vi "Text control 1 v0.4.vi"() -> ()   [LabVIEW 2016]
panel:
  in  "Sample I - Probe 4 (Disabled)":u32(ring)=3 items=["SMU1  ", "SMU2  ", "SMU3  ", "SMU4  ", "SMU5  ", "SMU6  ", "VSU1  ", "VSU2  "]
  in  "Sample I - Source/Common":u32(ring) items=["SMU1  ", "SMU2  ", "SMU3  ", "SMU4  ", "SMU5  ", "SMU6  ", "VSU1  ", "VSU2  "]
  in  "Sample I - Probe 3 (Disabled)":u32(ring)=2 items=["SMU1  ", "SMU2  ", "SMU3  ", "SMU4  ", "SMU5  ", "SMU6  ", "VSU1  ", "VSU2  "]
  in  "Sample I - Drain/Gate":u32(ring)=1 items=["SMU1  ", "SMU2  ", "SMU3  ", "SMU4  ", "SMU5  ", "SMU6  ", "VSU1  ", "VSU2  "]
  in  "Sample - Probe 4":u32(ring)=3 items=["SMU1  ", "SMU2  ", "SMU3  ", "SMU4  ", "SMU5  ", "SMU6  ", "VSU1  ", "VSU2  "]
  in  "Sample - Source/Common":u32(ring) items=["SMU1  ", "SMU2  ", "SMU3  ", "SMU4  ", "SMU5  ", "SMU6  ", "VSU1  ", "VSU2  "]
  in  "Sample - Gate":u32(ring)=2 items=["SMU1  ", "SMU2  ", "SMU3  ", "SMU4  ", "SMU5  ", "SMU6  ", "VSU1  ", "VSU2  "]
  in  "Sample - Drain":u32(ring)=1 items=["SMU1  ", "SMU2  ", "SMU3  ", "SMU4  ", "SMU5  ", "SMU6  ", "VSU1  ", "VSU2  "]
  in  "VSU2 Stress - Source/Common":u32(ring) items=["SMU1  ", "SMU2  ", "SMU3  ", "SMU4  ", "SMU5  ", "SMU6  ", "VSU1  "]
  in  "Stress I - Source/Common":u32(ring) items=["SMU1  ", "SMU2  ", "SMU3  ", "SMU4  ", "SMU5  ", "SMU6  ", "VSU1  ", "VSU2  "]
  in  "Stress I - Drain/Gate":u32(ring)=1 items=["SMU1  ", "SMU2  ", "SMU3  ", "SMU4  ", "SMU5  ", "SMU6  ", "VSU1  ", "VSU2  "]
  in  "Stress V - Source/Common":u32(ring) items=["SMU1  ", "SMU2  ", "SMU3  ", "SMU4  ", "SMU5  ", "SMU6  ", "VSU1  ", "VSU2  "]
  in  "Stress V - Gate":u32(ring)=2 items=["SMU1  ", "SMU2  ", "SMU3  ", "SMU4  ", "SMU5  ", "SMU6  ", "VSU1  ", "VSU2  "]
  in  "Stress V - Drain":u32(ring)=1 items=["SMU1  ", "SMU2  ", "SMU3  ", "SMU4  ", "SMU5  ", "SMU6  ", "VSU1  ", "VSU2  "]
  in  "FPP - Source":u32(ring)=6 items=["SMU1  ", "SMU2  ", "SMU3  ", "SMU4  ", "SMU5  ", "SMU6  ", "VSU1  ", "VSU2  "]
  in  "FPP - Probe 2":u32(ring)=3 items=["SMU1  ", "SMU2  ", "SMU3  ", "SMU4  ", "SMU5  ", "SMU6  ", "VSU1  ", "VSU2  "]
  in  "FPP - Probe 1":u32(ring) items=["SMU1  ", "SMU2  ", "SMU3  ", "SMU4  ", "SMU5  ", "SMU6  ", "VSU1  ", "VSU2  "]
  in  "FPP - Gate":u32(ring)=2 items=["SMU1  ", "SMU2  ", "SMU3  ", "SMU4  ", "SMU5  ", "SMU6  ", "VSU1  ", "VSU2  "]
  in  "FPP - Drain":u32(ring)=1 items=["SMU1  ", "SMU2  ", "SMU3  ", "SMU4  ", "SMU5  ", "SMU6  ", "VSU1  ", "VSU2  "]
  in  "Pulsed Stress V - Gate":u32(ring)=2 items=["SMU1  ", "SMU2  ", "SMU3  ", "SMU4  ", "SMU5  ", "SMU6  ", "VSU1  ", "VSU2  "]
  in  "Pulsed Stress V - Source/Common":u32(ring) items=["SMU1  ", "SMU2  ", "SMU3  ", "SMU4  ", "SMU5  ", "SMU6  ", "VSU1  ", "VSU2  "]
  in  "Pulsed Stress V - Drain":u32(ring)=1 items=["SMU1  ", "SMU2  ", "SMU3  ", "SMU4  ", "SMU5  ", "SMU6  ", "VSU1  ", "VSU2  "]
  in  "Pulsed Stress V - Vextra":u32(ring)=7 items=["SMU1  ", "SMU2  ", "SMU3  ", "SMU4  ", "SMU5  ", "SMU6  ", "VSU1  ", "VSU2  "]
  in  "Pulsed Stress V - Probe 4":u32(ring)=3 items=["SMU1  ", "SMU2  ", "SMU3  ", "SMU4  ", "SMU5  ", "SMU6  ", "VSU1  ", "VSU2  "]
  in  "Transfer/Output - Probe 4":u32(ring)=3 items=["SMU1  ", "SMU2  ", "SMU3  ", "SMU4  ", "SMU5  ", "SMU6  ", "VSU1  ", "VSU2  "]
  in  "Transfer/Output - Source/Common":u32(ring) items=["SMU1  ", "SMU2  ", "SMU3  ", "SMU4  ", "SMU5  ", "SMU6  ", "VSU1  ", "VSU2  "]
  in  "Transfer/Output - Gate":u32(ring)=2 items=["SMU1  ", "SMU2  ", "SMU3  ", "SMU4  ", "SMU5  ", "SMU6  ", "VSU1  ", "VSU2  "]
  in  "Transfer/Output - Drain":u32(ring)=1 items=["SMU1  ", "SMU2  ", "SMU3  ", "SMU4  ", "SMU5  ", "SMU6  ", "VSU1  ", "VSU2  "]
  in  "Panel Controls 2":T1={"Emergency Stop"=refnum, "TransGraph Max"=1e-05, "Text/Graph (text=false)"=TRUE, "TransGraph Min"=1e-11} {"TransGraph Min" format="%.2e"; "TransGraph Max" format="%.2e"}
  out "Currently running:":string="#output s 0 0 0 -0.008 0.008 0.002"
  in  "Lines left to run:":string
  in  "Standby":T2
  in  "Full Reset":bool
  in  "SMU4":cluster{"on/off":bool, "Voltage":dbl} {"Voltage" min=-100.0 max=100.0 format="%.2f"}
  in  "Source/Drain\nRange":u8(slide)=6 max=11 scale=0.0..11.0
  in  "Source/Drain\nRange mode":u16(ring) items=["Auto", "Limited", "Fixed"]
  in  "Gate Range":u8(slide)=6 max=11 scale=0.0..11.0
  in  "Gate Range\nmode":u16(ring) items=["Auto", "Limited", "Fixed"]
  in  "Gate":T3={"Gate Start"=0.0, "Gate Stop"=2.0, "Gate Step (linear only)"=1.0, "Gate Compliance"=0.0001, "Gate PComp"=0.0, "Range mode"=0, "Range"=6} {"Range" max=11 scale=0.0..11.0; "Range mode" items=["Auto", "Limited", "Fixed"]; "Gate PComp" format="%^.2e"; "Gate Compliance" format="%^.2e"; "Gate Step (linear only)" format="%^.4e"; "Gate Stop" format="%^.4e"; "Gate Start" format="%^.4e"}
  in  "Drain 2":T4={"Drain Start"=0.0, "Drain Stop"=2.0, "Drain Compliance"=0.0001, "Drain Step"=1.0, "Drain PComp"=0.0, "Range mode"=0, "Range"=6} {"Range" max=11 scale=0.0..11.0; "Range mode" items=["Auto", "Limited", "Fixed"]; "Drain PComp" format="%^.2e"; "Drain Step" format="%^.4e"; "Drain Compliance" format="%^.2e"; "Drain Stop" format="%^.4e"; "Drain Start" format="%^.4e"}
  in  "Timings 2":T5={"integration time"=0, "Short/Long integration time"=0.00064, "hold time (sec)"=0.0, "delay time (sec)"=0.0, "Step Time (0 disables)"=0.0, "sweep method"=0, "Pulse period"=0.005, "Base voltage"=0.0, "Pulse width"=0.0005} {"Pulse width" min=0.0005 max=0.1 step=0.0001 format="%.4f"; "Base voltage" format="%^.4e"; "Pulse period" min=0.005 max=1.0 step=0.0001 format="%.4f"; "sweep method" items=["Continuous", "Pulsed"]; "Step Time (0 disables)" format="%.2f"; "delay time (sec)" format="%.4f"; "hold time (sec)" format="%.4f"; "Short/Long integration time" format="%^.0e"; "integration time" scale=0.0..2.0}
  in  "Panel Controls":T6={"Emergency Stop"=refnum, "TransGraph Max"=1e-05, "Text/Graph (text=false)"=TRUE} {"TransGraph Max" format="%.2e"}
  in  "Interrupt run":bool
  in  "Drain: Compliance":dbl=0.001 format="%.8f"
  in  "Gate: Compliance":dbl=0.001 format="%.8f"
  out "Path":path=path "C:/users/rlp38/09Apr2009LTtesting/test2.txt"
  in  "hold time /s":dbl format="%.2f"
  in  "delay time /s":dbl format="%.2f"
  in  "integration time":u32(slide)=1 max=2 step=1 scale=0.0..2.0
  in  "Integration time (short)":dbl=0.0019 min=8e-05 max=0.0019 step=8e-05 format="%^.0e"
  in  "Integration time (long)":dbl=0.32 min=0.04 max=2.0 step=0.02 format="%.2f"
  in  "Step delay /s":dbl format="%.2f"
  in  "Program":string="#pulsedstressV d 0.03 20 0 0.5 0.0827 5\n#\n#itime l 0.32\n#gaterangemode a\n#drainrangemode a\n#pulsed on 0.05 0 0.02\n#transfer d -10 40 1 5 40 35\n#transfer d -10 40 1 5 40 35\n#transfer d -10 40 1 5 40 35\n#output d 0 40 20 0 40 1\n#\n#\n#sample 1 0.008 221 6 0.003\n#samplei 400e-6 200 6 0.002 0.1\n#vsu2pulse -10 4\n#\n#stressV 0.016 0.03 2e-4 0.1e-3 11\n#stressI 220e-7 0.08 15\n#transfer s -1 1 0.5 -0.005 0.005 0.005\n#output s 0 0 0 -0.008 0.008 0.002\n"
  # "SMUs"
  # "Syntax:\nitime [s|m|l] time(sec): [s|m|l] determines the integration time setting (small|medium|long) and time sets the value.\nNOTE: The value of the integration time has to be within the range allowed by its category (s|m|l), otherwise, the closest value will be used. (e.g. if the category is set to short but the time value is very long, the actual value used will be the maximum short integration time.\nIntegration times:\n    Short: Default: 640 us. Range: 8E-5 - 1.92E-3 seconds.\n    Medium: Fixed at 1 NPL cycle (0.02 seconds).\n    Long: Default: 16 NPL cycles (0.32 seconds). Range: 2-100 NPL cycles (0.04 seconds - 2 seconds).\ngaterangemode [a|l|f]\ndrainrangemode [a|l|f]\npulsed [on|off] PulsePeriod(sec) PulseBaseVoltage PulseONWidth(sec)\nstandby [on l off]\nwait NumMilliseconds\nwait-min NumMinutes\n# texthere = comment\ntransfer [s|d] VgStart VgStop VgStep VdStart VdStop VdStep\noutput [s|d] VgStart VgStop VgStep VdStart VdStop VdStep\nsample Vg Vd NumSamples Time(s) SampleInterval(s)\nsamplei Idg NumSamples Time(s) SampleInterval(s) VDGcompliance\n# if in doubt use SampleInterval(s) = 0.004\nstressV VG VD IGcompliance IDcompliance Duration(sec)\nstressI IDG VDGcompliance Duration(sec)\nvsu2pulse Bias Duration(s)\npulsedstressV [s|d] VEstop VgON VgOFF Period(s) PulseONwidth(s) Vd\nsample-fpp Vg Vd NumSamples Time\nresample-fpp Vg Vd\ntransfer-fpp [s|d] VgStart VgStop VgStep VdStart VdStop VdStep\noutput-fpp [s|d] VgStart VgStop VgStep VdStart VdStop VdStep"
  # "100 samples is approx 13s with medium integration"
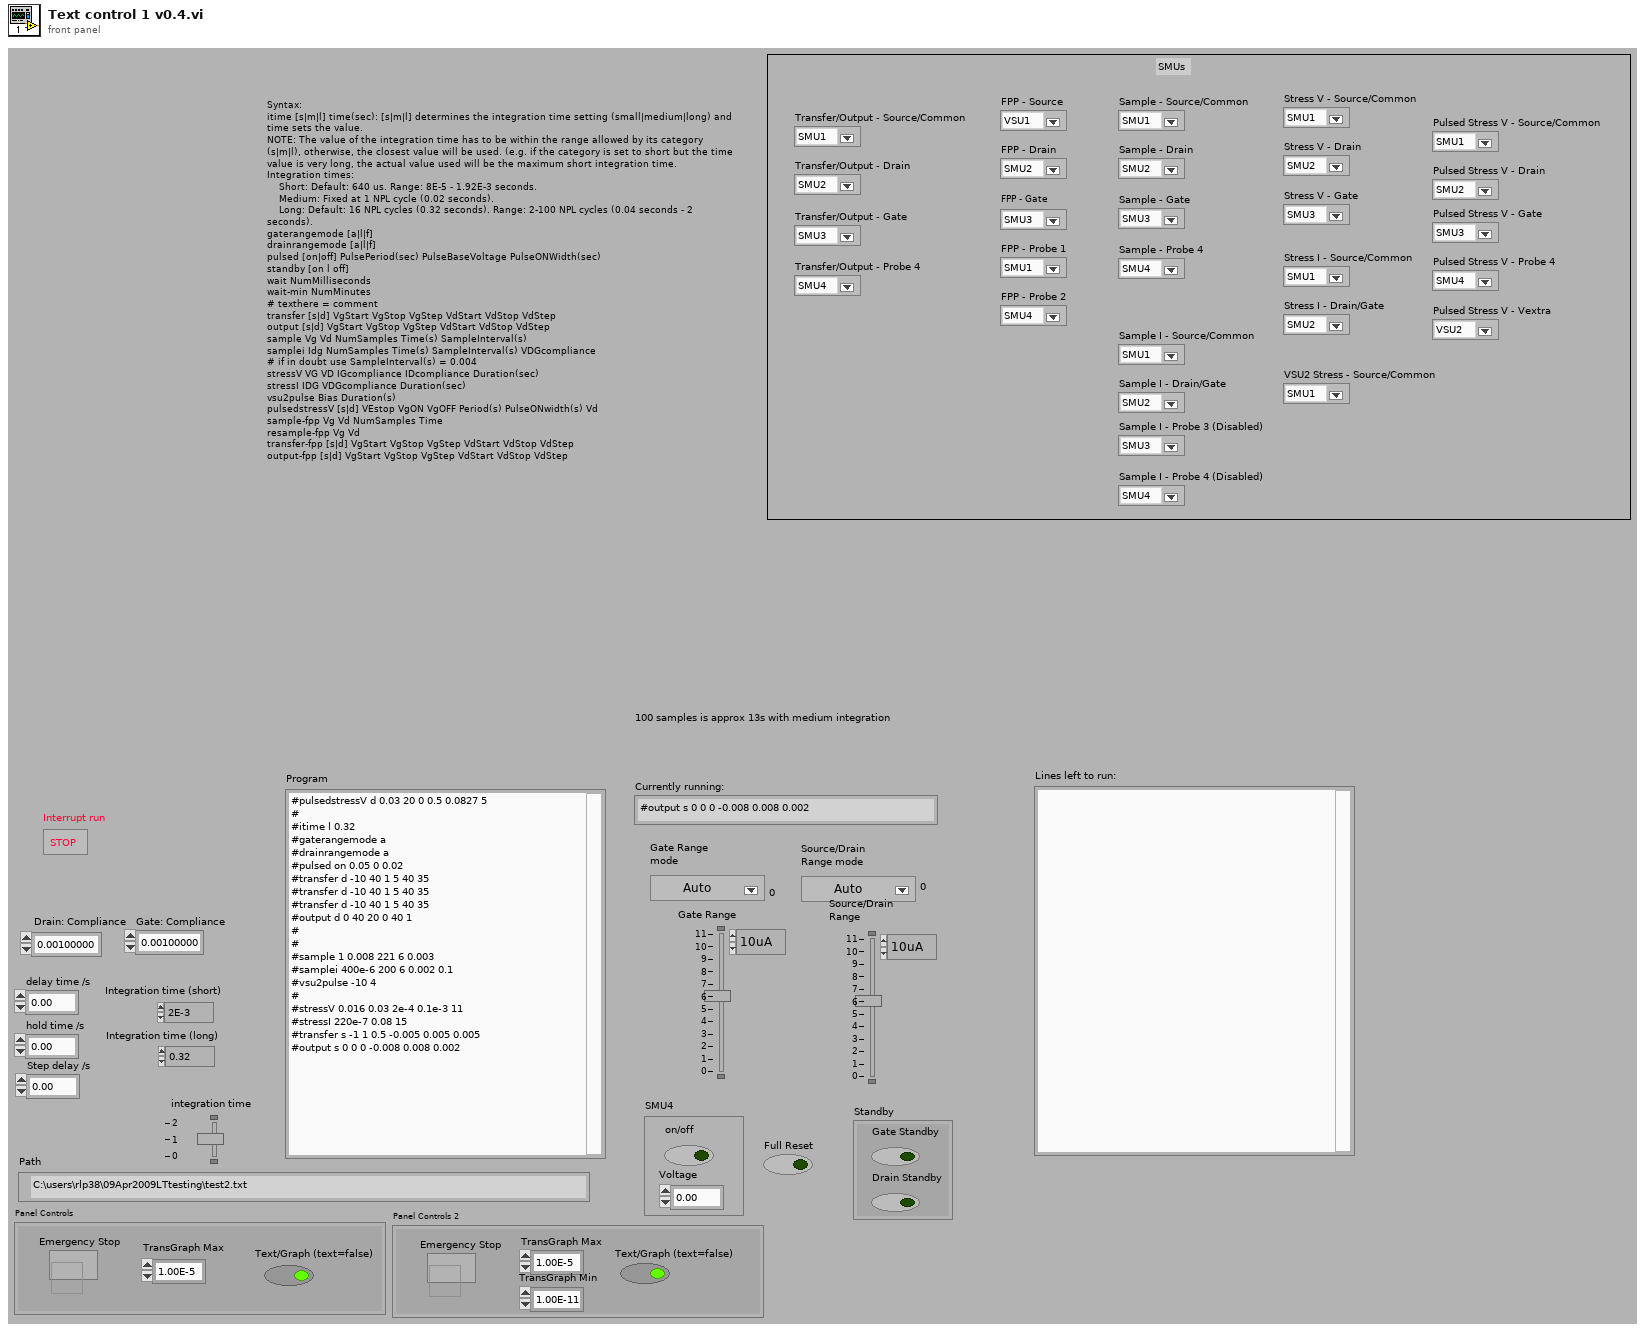
[diagram p1: front panel]
types:
  T1 = cluster{"Emergency Stop":refnum<vi>, "TransGraph Max":dbl, "Text/Graph (text=false)":bool, "TransGraph Min":dbl}
  T2 = cluster{"Gate Standby":bool, "Drain Standby":bool}
  T3 = cluster{"Gate Start":dbl, "Gate Stop":dbl, "Gate Step (linear only)":dbl, "Gate Compliance":dbl, "Gate PComp":dbl, "Range mode":u16, "Range":u8}
  T4 = cluster{"Drain Start":dbl, "Drain Stop":dbl, "Drain Compliance":dbl, "Drain Step":dbl, "Drain PComp":dbl, "Range mode":u16, "Range":u8}
  T5 = cluster{"integration time":u32, "Short/Long integration time":dbl, "hold time (sec)":dbl, "delay time (sec)":dbl, "Step Time (0 disables)":dbl, "sweep method":u16, "Pulse period":dbl, "Base voltage":dbl, "Pulse width":dbl}
  T6 = cluster{"Emergency Stop":refnum<vi>, "TransGraph Max":dbl, "Text/Graph (text=false)":bool}
  T7 = enum16{"open", "replace", "create", "open or create", "replace or create", "replace or create with confirmation"}
  T8 = cluster{"V2 Start":dbl, "V2 Step":dbl, "Number of points":i32}
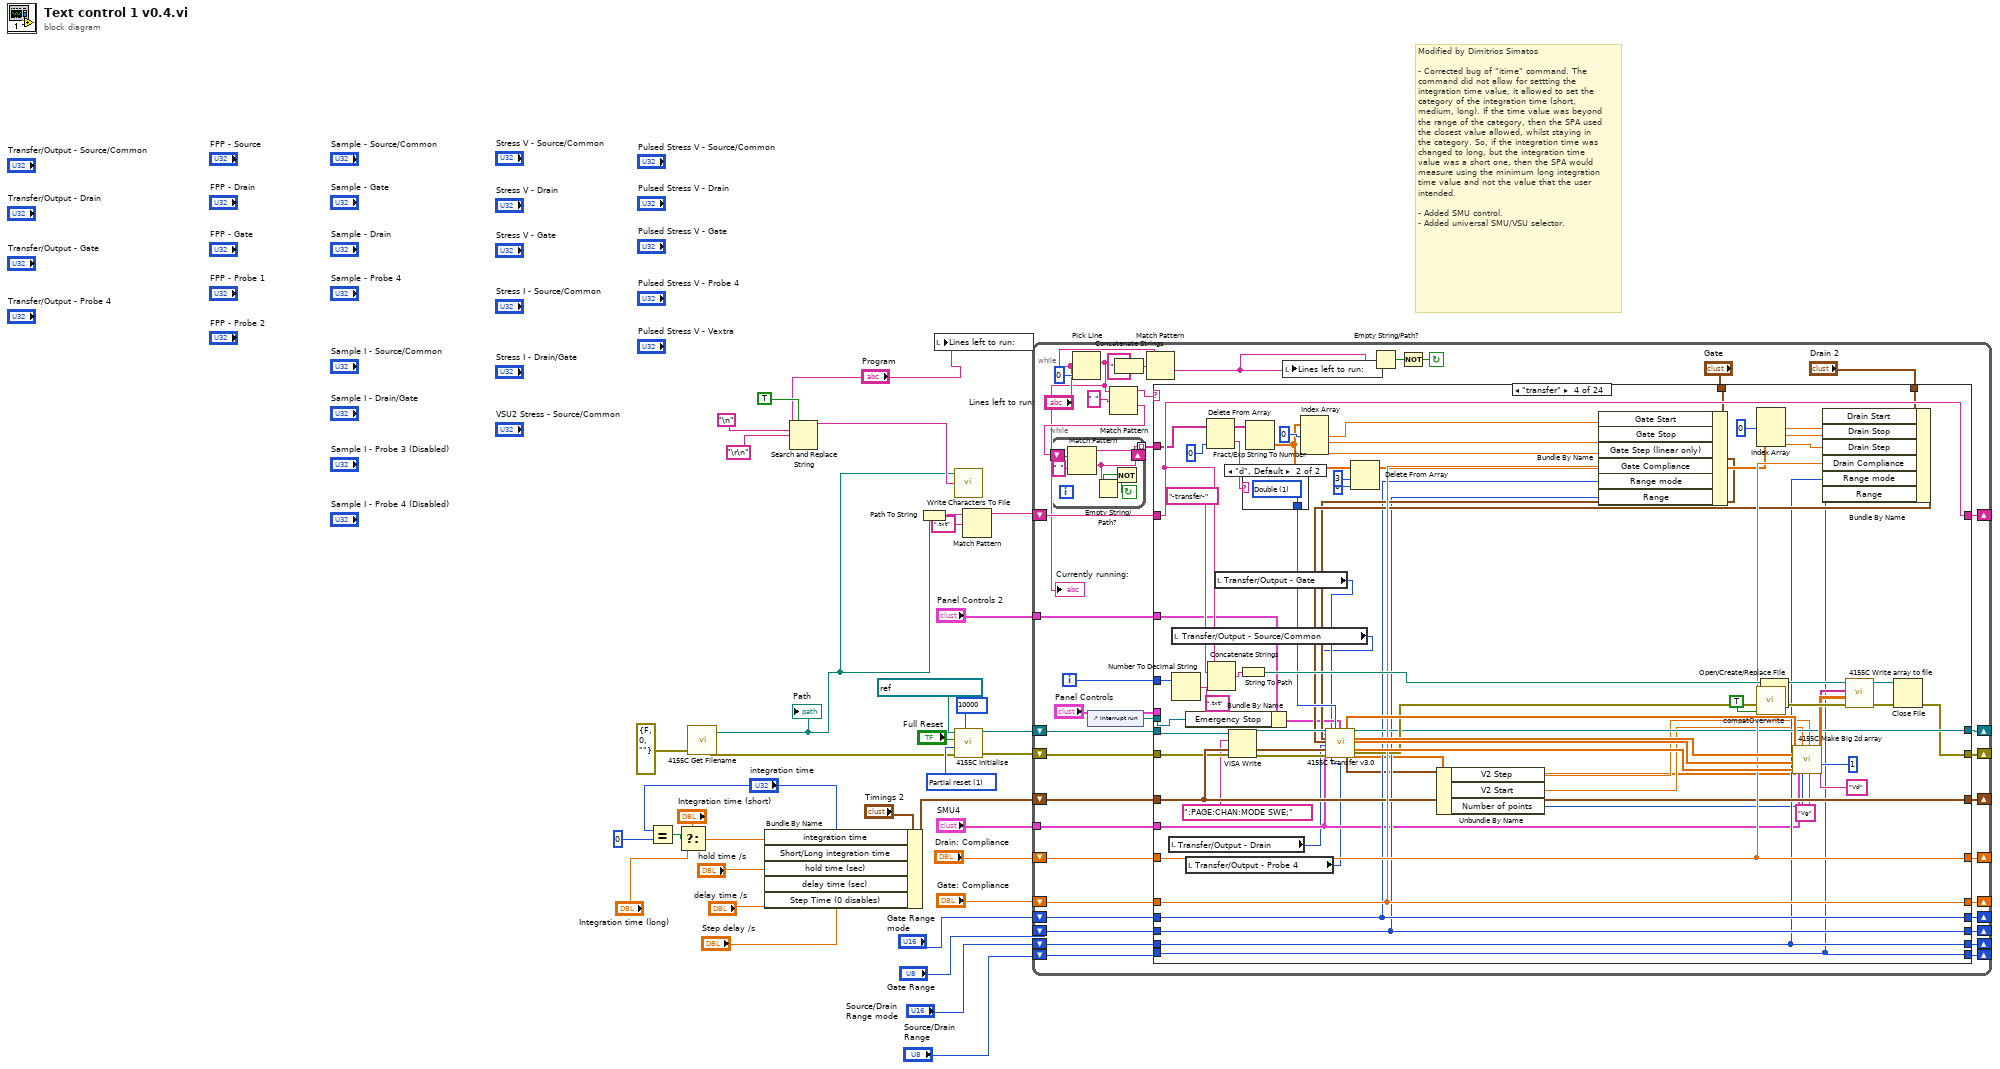
[diagram p0: block diagram]
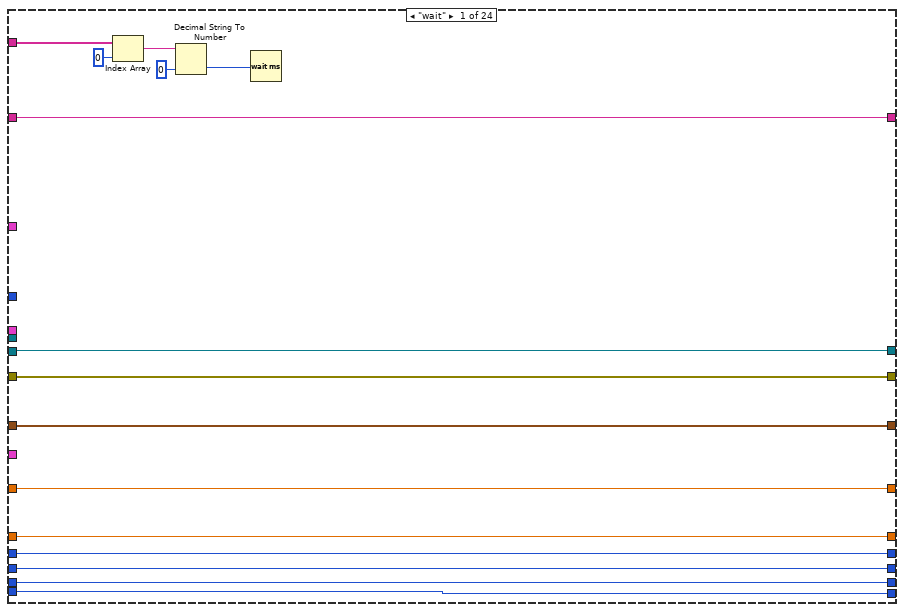
[diagram p2: hidden frame]
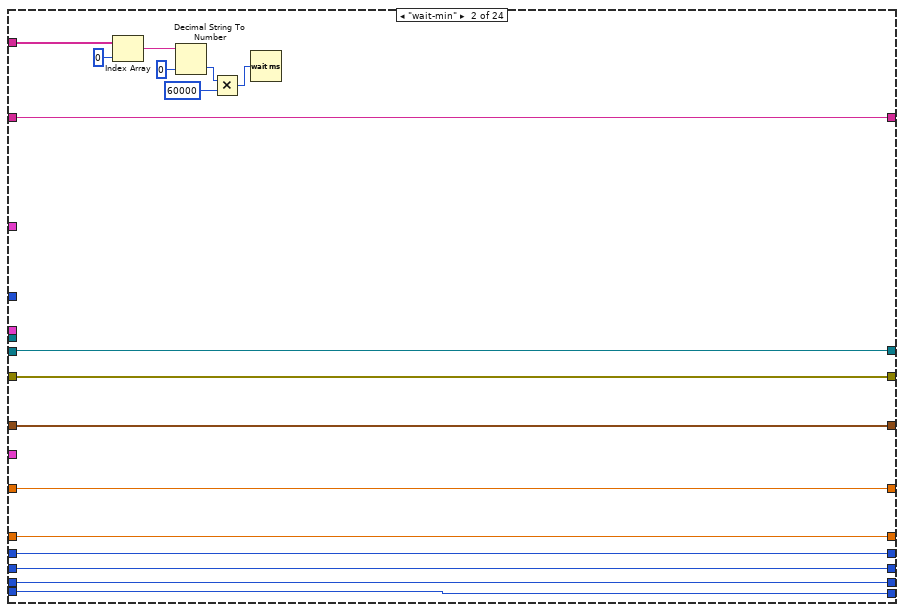
[diagram p3: hidden frame]
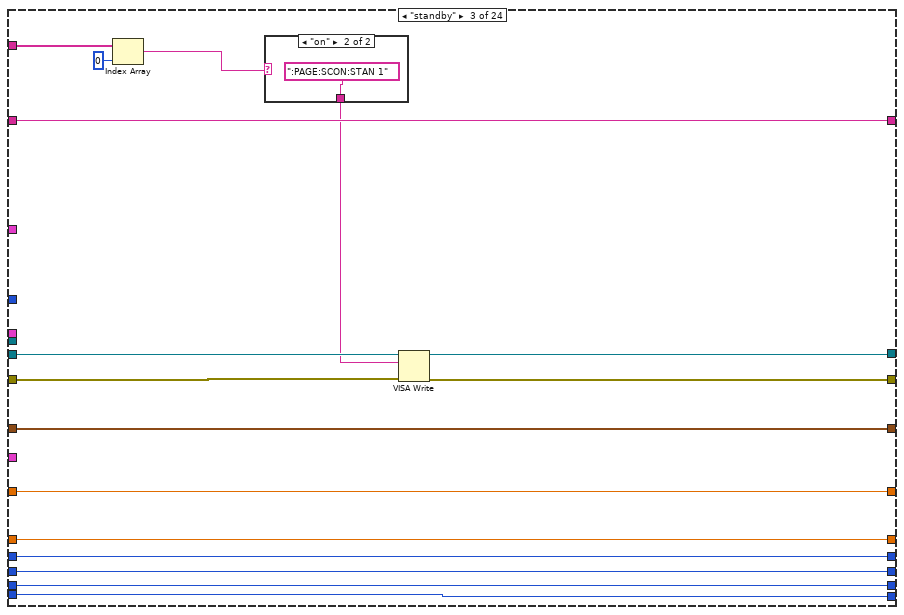
[diagram p4: hidden frame]
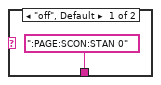
[diagram p5: hidden frame]
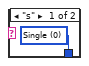
[diagram p6: hidden frame]
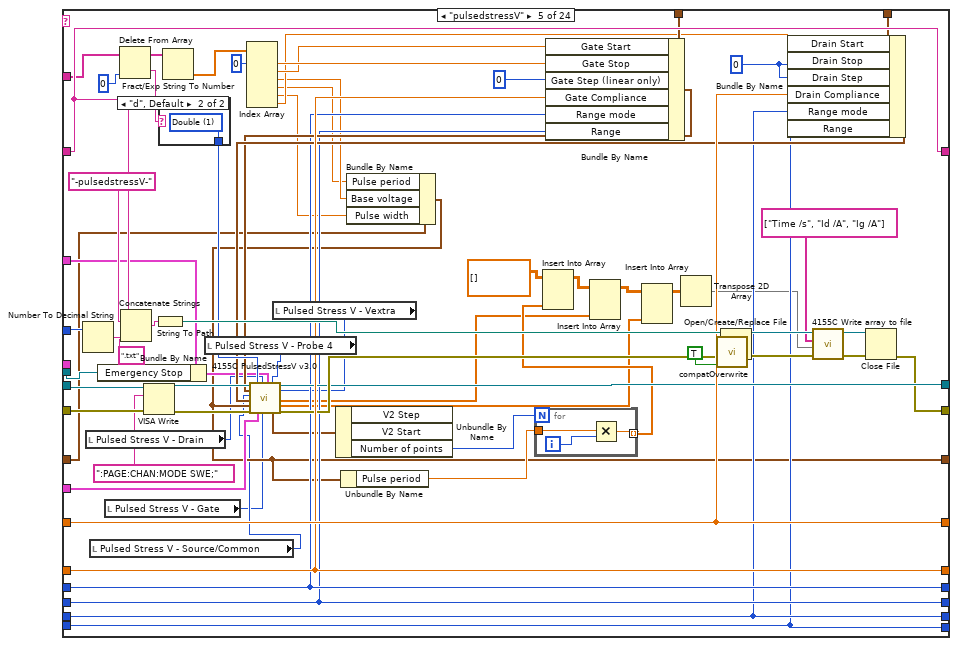
[diagram p7: hidden frame]
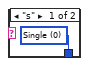
[diagram p8: hidden frame]
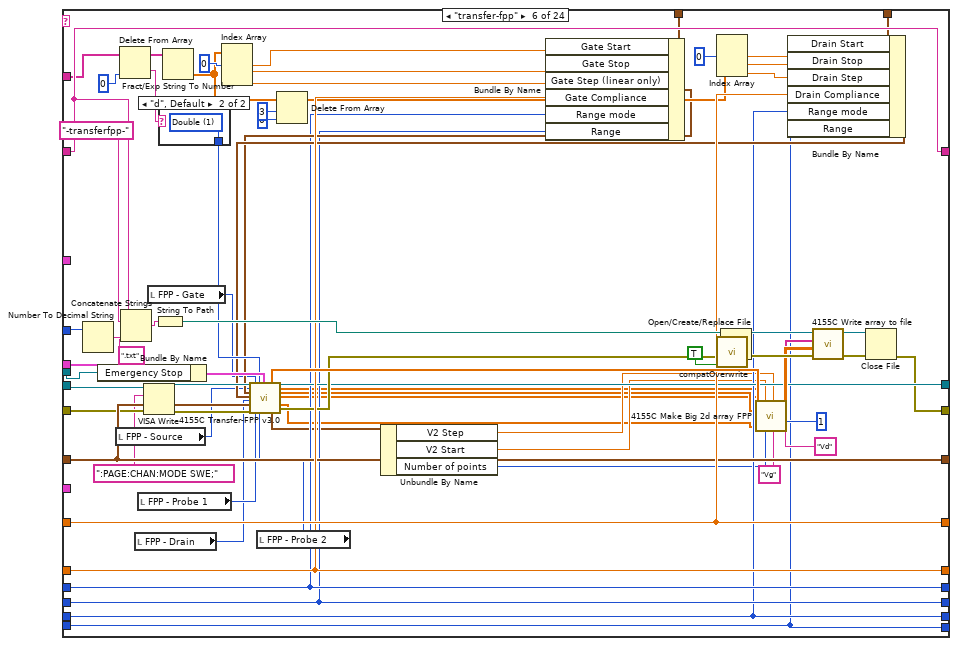
[diagram p9: hidden frame]
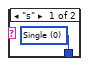
[diagram p10: hidden frame]
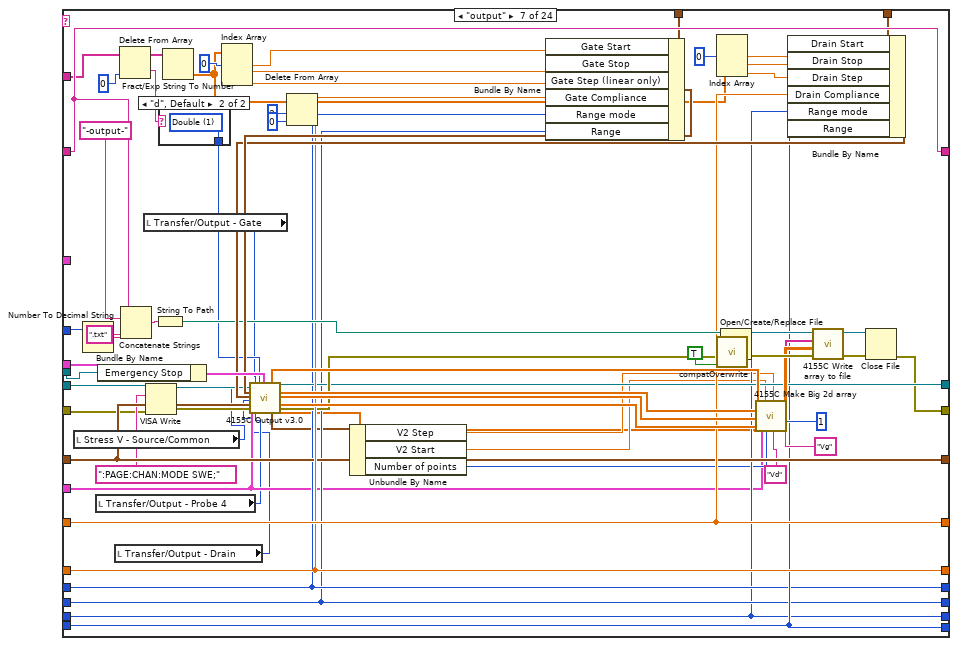
[diagram p11: hidden frame]
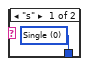
[diagram p12: hidden frame]
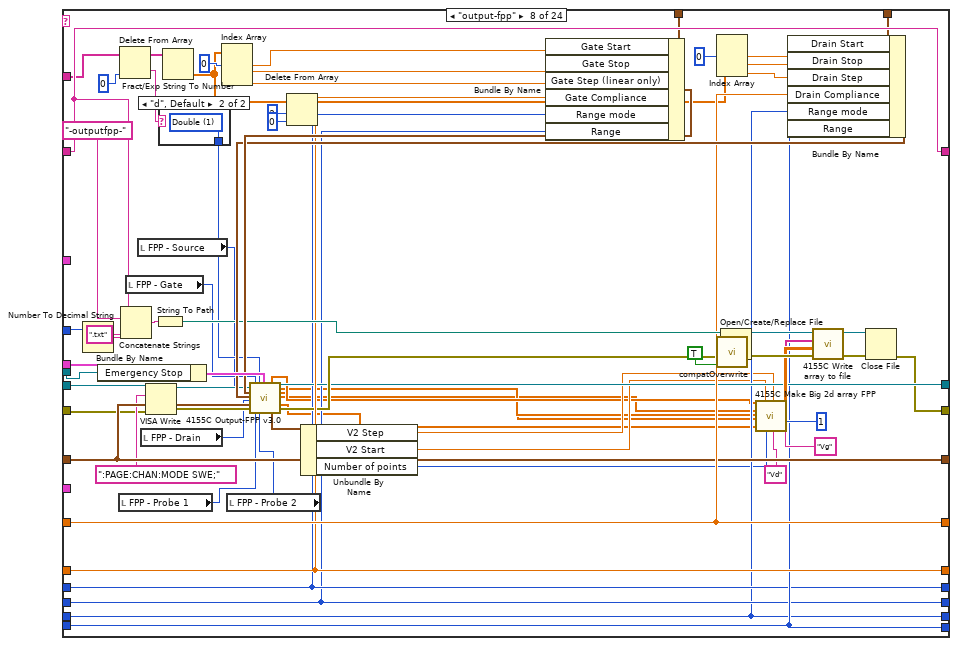
[diagram p13: hidden frame]
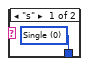
[diagram p14: hidden frame]
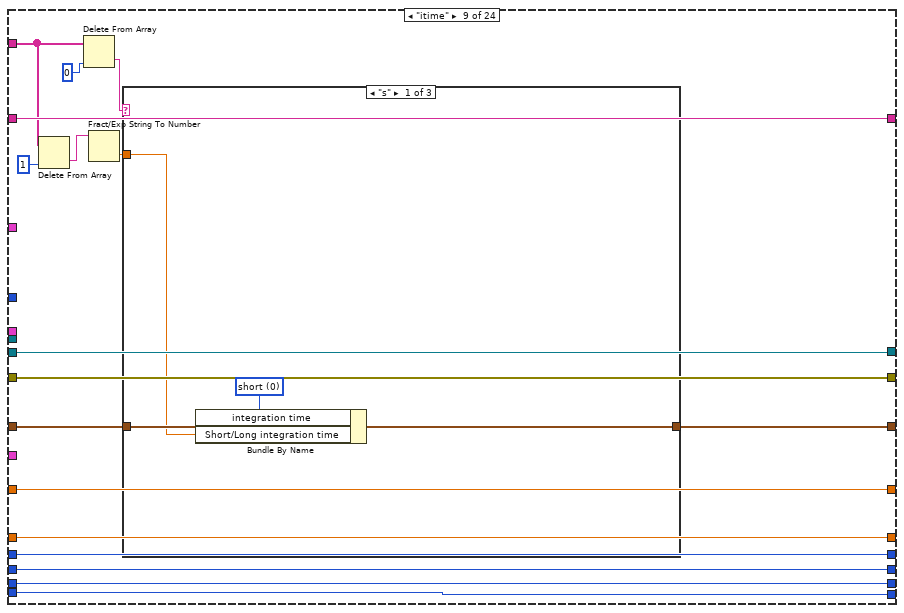
[diagram p15: hidden frame]
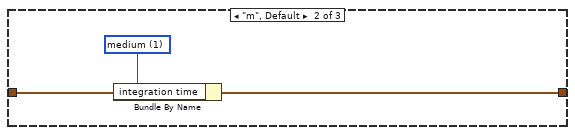
[diagram p16: hidden frame]
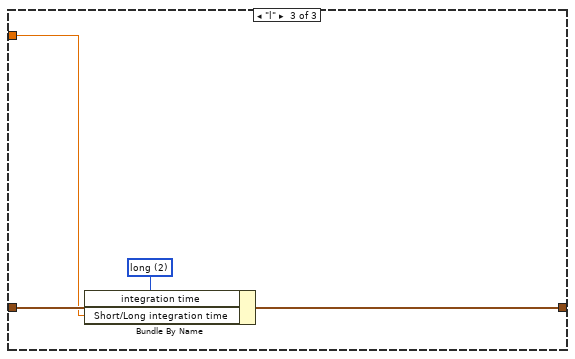
[diagram p17: hidden frame]
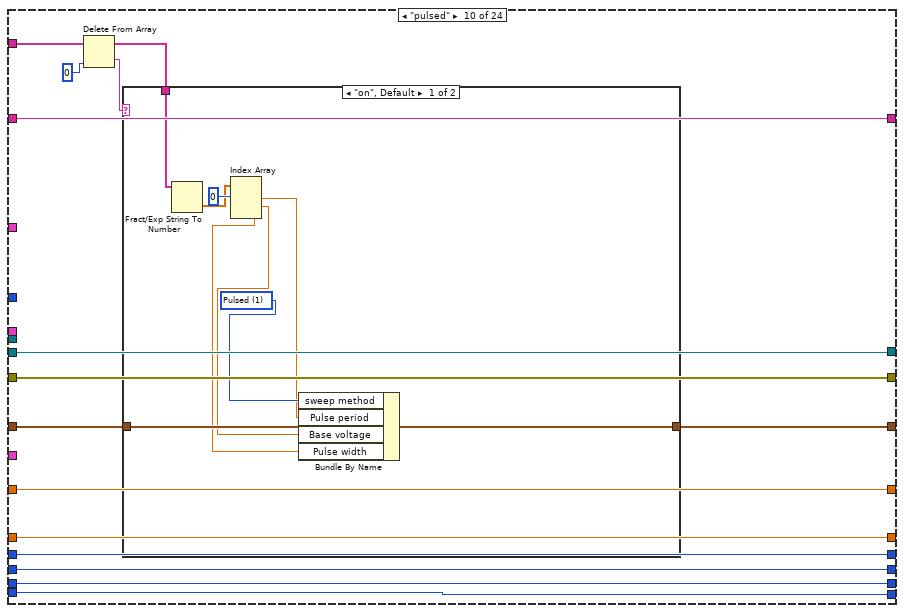
[diagram p18: hidden frame]
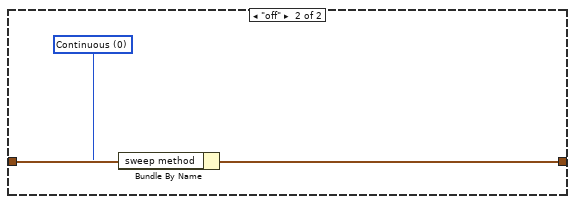
[diagram p19: hidden frame]
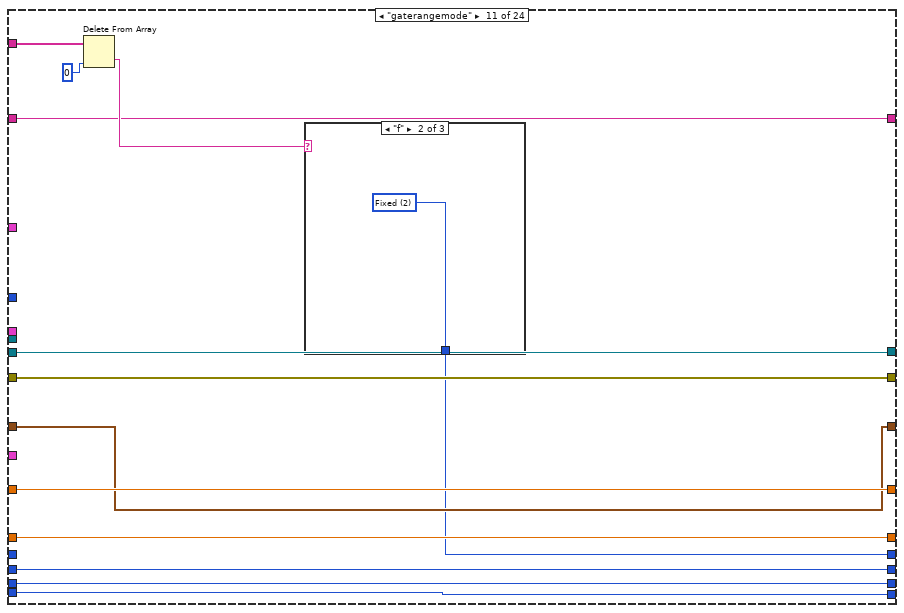
[diagram p20: hidden frame]
diagram:
  w27 = u16 1 items=["Reset All", "Partial reset"] ("Type of reset")
  # "Modified by Dimitrios Simatos\n\n- Corrected bug of \"itime\" command. The command did not allow for settting the integration time value, it allowed to set the category of the integration time (short, medium, long). If the time value was beyond the range of the category, then the SPA used the closest value allowed, whilst staying in the category. So, if the integration time was changed to long, but the integration time value was a short one, then the SPA would measure using the minimum long integration time value and not the value that the user intended.\n\n- Added SMU control.\n- Added universal SMU/VSU selector."
  n1 = Equal?(x="integration time", y=u32 0) -> (x = y?=w31:bool)
  n2 = Select(t="Integration time (short)", s=w31, f="Integration time (long)") -> (s? t:f=w35:dbl)
  n3 = call "4155C Get Filename.vi"("error in (no error)"=errorcluster {"status"=FALSE, "code"=0, "source"=""}) -> ("error out"=w22:errorcluster, "path"=w6:path)  [unwired: 2 in, 1 out]
  "Path" <- w6
  n4 = Bundle By Name(cluster="Timings 2", "integration time"="integration time", "Short/Long integration time"=w35, "hold time (sec)"="hold time /s", "delay time (sec)"="delay time /s", "Step Time (0 disables)"="Step delay /s") -> (w19:T5)
  n5 = Search and Replace String(replace all?=TRUE ("replace all? (F)"), input string="Program", search string="\n", replace string="\r\n") -> (result string=w9:string)  [unwired: 4 in, 3 out]
  n6 = Path To String(path=w6) -> (string=w5:string)
  n7 = local write "Lines left to run:"("Program") -> ()
  n8 = call <vilib>:"Write Characters To File.vi"("character string"=w9, "file path (dialog if empty)"=w6) -> ()  [unwired: 3 in, 1 out]
  n9 = call "4155C Initialise.vi"("VISA resource name in"=refnum<visa-resource-name> "GPIB0::14::INSTR", "Reset"="Full Reset", "Type of reset"=w27, "error in (no error)"=w22, "VISA Timeout Value"=u32 10000) -> ("VISA Resource Name out"=w21:refnum<visa-resource-name>, "error out"=w20:errorcluster)
  n10 = Match Pattern(string=w5, regular expression=".txt") -> (before substring=w4:string)  [unwired: 1 in, 3 out]
  n11 = while {
    tunnel: "SMU4" -> [w41]
    shift-left: "Source/Drain\nRange" -> [w46]
    shift-right: [w42] -> _
    shift-left: "Source/Drain\nRange mode" -> [w47]
    shift-right: [w43] -> _
    shift-left: "Gate Range" -> [w48]
    shift-right: [w44] -> _
    shift-left: "Gate Range\nmode" -> [w49]
    shift-right: [w45] -> _
    shift-left: "Gate: Compliance" -> [w61]
    shift-right: [w55] -> _
    shift-left: "Drain: Compliance" -> [w62]
    shift-right: [w56] -> _
    shift-left: w19 -> [w63]
    shift-right: [w57] -> _
    shift-left: w20 -> [w64]
    shift-right: [w58] -> _
    shift-left: w21 -> [w65]
    shift-right: [w59] -> _
    shift-left: w4 -> [w66]
    shift-right: [w54] -> _
    tunnel: "Panel Controls 2" -> [w37]
    i -> [w60]
    stop <- w74 continue-if-true
    n12 = Pick Line(multi-line string="Lines left to run:", line index=0) -> (output string=w38:string)  [unwired: 1 in]
    "Currently running:" <- w38
    n13 = control-ref of="Interrupt run"() -> (w53:refnum<vi>)
    n14 = Match Pattern(string=w38, regular expression=" ") -> (before substring=w69:string, after substring=w68:string)  [unwired: 1 in, 2 out]
    n15 = while {
      tunnel: [w76] -> w67 mode=indexing
      shift-left: w68 -> [w78]
      shift-right: [w77] -> _
      stop <- w80 continue-if-true
      n16 = Match Pattern(string=w78, regular expression=" ") -> (before substring=w76:string, after substring=w77:string)  [unwired: 1 in, 2 out]
      n17 = Empty String/Path?(string/path=w77) -> (empty?=w81:bool)
      n18 = Not(x=w81) -> (.not. x?=w80:bool)
    }
    n19 = Concatenate Strings(w38, "\n" ("Substring")) -> (w72:string)
    n20 = Match Pattern(string="Lines left to run:", regular expression=w72) -> (after substring=w39:string)  [unwired: 1 in, 3 out]
    n21 = case shown="\"transfer\"" w69 {
      tunnel: w67 -> [w96 w113 w129 w178 w256 w327 w395 w472 w500 w538 w563 w586 w605 w617 _ _ w716 w778 _ w841 w884 w924 w996 w1055]
      tunnel: w66 -> [w91 w109 w127 w186 w263 w335 w403 w480 w502 w527 w555 w579 w599 w610 w627 w665 w694 w760 w790 w828 w871 w912 w990 w1051]
      tunnel: w65 -> [w90 w108 w118 w156 w247 w304 w371 w448 w503 w528 w556 w580 w600 w611 w632 w668 w723 w785 w794 w848 w891 w931 w1003 w1008]
      tunnel: w64 -> [w89 w107 w117 w155 w246 w303 w368 w445 w504 w529 w557 w581 w601 w612 w631 w637 w722 w784 w793 w847 w890 w930 w1002 w1007]
      tunnel: w63 -> [w88 w106 w126 w182 w221 w331 w399 w476 w512 w537 w554 w578 w598 w609 w630 w661 w685 w752 w799 w821 w864 w905 w989 w1050]
      tunnel: w62 -> [w87 w105 w125 w184 w261 w333 w401 w478 w511 w536 w562 w585 w604 w616 w629 w646 w721 w783 w802 w846 w889 w929 w1001 w1060]
      tunnel: w61 -> [w86 w104 w124 w183 w260 w332 w400 w477 w510 w535 w561 w584 w603 w615 w628 w647 w695 w761 w801 w829 w872 w913 w991 w1052]
      tunnel: w60 -> [_ _ _ w187 w264 w336 w404 w481 _ _ _ _ _ _ _ w663 w720 w782 _ w845 w888 w928 w1000 w1059]
      tunnel: [w90 w108 w116 w180 w258 w329 w397 w474 w503 w528 w556 w580 w600 w611 w632 w668 w686 w733 w792 w822 w865 w906 w941 w1010] -> w59
      tunnel: [w89 w107 w115 w179 w257 w328 w396 w473 w504 w529 w557 w581 w601 w612 w631 w636 w696 w734 w791 w830 w873 w914 w940 w1009] -> w58
      tunnel: [w88 w106 w126 w182 w217 w331 w399 w476 w505 w530 w554 w578 w598 w609 w630 w661 w685 w752 w799 w821 w864 w905 w989 w1050] -> w57
      tunnel: [w87 w105 w125 w184 w261 w333 w401 w478 w511 w536 w562 w585 w604 w616 w629 w646 w721 w783 w802 w846 w889 w929 w1001 w1060] -> w56
      tunnel: [w86 w104 w124 w183 w260 w332 w400 w477 w510 w535 w561 w584 w603 w615 w628 w647 w695 w761 w801 w829 w872 w913 w991 w1052] -> w55
      tunnel: [w91 w109 w127 w186 w263 w335 w403 w480 w502 w527 w555 w579 w599 w610 w627 w665 w694 w760 w790 w828 w871 w912 w990 w1051] -> w54
      tunnel: w53 -> [_ _ _ w195 w268 w341 w412 w485 _ _ _ _ _ _ _ _ w691 w757 _ w827 w870 w911 w961 w1026]
      tunnel: "Gate" -> [_ _ _ w165 w250 w314 w382 w459 _ _ _ _ _ _ _ _ _ _ _ _ _ _ _ _]
      tunnel: "Drain 2" -> [_ _ _ w164 w249 w313 w381 w458 _ _ _ _ _ _ _ _ _ _ _ _ _ _ _ _]
      tunnel: "Panel Controls" -> [_ _ _ _ _ w312 w380 w457 _ _ _ _ _ _ _ _ _ _ _ _ _ _ _ _]
      tunnel: w49 -> [w85 w103 w123 w149 w240 w297 w366 w443 w509 w534 _ w577 w597 w608 w626 w648 w681 w748 w795 w817 w860 w901 w985 w1046]
      tunnel: w48 -> [w84 w102 w122 w148 w239 w296 w365 w442 w508 w533 w560 _ w588 w614 w625 w649 w682 w749 w796 w818 w861 w902 w986 w1047]
      tunnel: w47 -> [w83 w101 w121 w147 w238 w295 w364 w441 w507 w532 w559 w583 w602 _ w624 w650 w683 w750 w797 w819 w862 w903 w987 w1048]
      tunnel: w46 -> [w82 w100 w120 w146 w237 w294 w367 w444 w506 w531 w558 w582 _ w613 w623 w651 w684 w751 w798 w820 w863 w904 w988 w1049]
      tunnel: [w85 w103 w123 w149 w240 w297 w366 w443 w509 w534 w553 w577 w597 w608 w626 w648 w681 w748 w795 w817 w860 w901 w985 w1046] -> w45
      tunnel: [w84 w102 w122 w148 w239 w296 w365 w442 w508 w533 w560 w569 w588 w614 w625 w649 w682 w749 w796 w818 w861 w902 w986 w1047] -> w44
      tunnel: [w83 w101 w121 w147 w238 w295 w364 w441 w507 w532 w559 w583 w602 w607 w624 w650 w683 w750 w797 w819 w862 w903 w987 w1048] -> w43
      tunnel: [w82 w100 w120 w146 w237 w294 w367 w444 w506 w531 w558 w582 w589 w613 w623 w651 w684 w751 w798 w820 w863 w904 w988 w1049] -> w42
      tunnel: w41 -> [_ _ _ w139 w233 _ w358 _ _ _ _ _ _ _ _ _ _ _ _ _ _ _ _ _]
      tunnel: w37 -> [_ _ _ w137 w232 _ _ _ _ _ _ _ _ _ _ _ _ _ _ _ _ _ _ _]
      frame "wait" {
        n22 = Index Array(array=w96, index=0 ("Index")) -> (element=w94:string)
        n23 = Decimal String To Number(string=w94, default (0L)=u32 0) -> (number=w93:u32)  [unwired: 1 in, 1 out]
        n24 = Wait (ms)(milliseconds to wait=w93) -> ()  [unwired: 1 out]
      }
      frame "wait-min" {
        n25 = Index Array(array=w113, index=0 ("Index")) -> (element=w111:string)
        n26 = Decimal String To Number(string=w111, default (0L)=u32 0) -> (number=w99:u32)  [unwired: 1 in, 1 out]
        n27 = Multiply(x=w99, y=u32 60000) -> (x*y=w98:u32)
        n28 = Wait (ms)(milliseconds to wait=w98) -> ()  [unwired: 1 out]
      }
      frame "standby" {
        n29 = Index Array(array=w129, index=0 ("Index")) -> (element=w119:string)
        n30 = case shown="\"on\"" w119 {
          tunnel: [":PAGE:SCON:STAN 0" ":PAGE:SCON:STAN 1"] -> w114
          frame "off", Default {
          }
          frame "on" {
          }
        }
        n31 = VISA Write(VISA resource name=w118, write buffer=w114, error in (no error)=w117) -> (VISA resource name out=w116:refnum<visa-resource-name>, error out=w115:errorcluster)  [unwired: 1 out]
      }
      frame "transfer" {
        n32 = local read "Transfer/Output - Drain"() -> (w133:u32)
        n33 = local read "Transfer/Output - Source/Common"() -> (w132:u32)
        n34 = Number To Decimal String(number=w187) -> (decimal integer string=w188:string)  [unwired: 1 in]
        n35 = Bundle By Name(cluster=w137, "Emergency Stop"=w195) -> (w138:T1)
        n36 = local read "Transfer/Output - Probe 4"() -> (w134:u32)
        n37 = Delete From Array(array=w178, index=0 ("Index")) -> (deleted portion=w176:string, array with subset deleted=w175:string[])  [unwired: 1 in]
        n38 = Concatenate Strings(w186, "-transfer-" ("Substring"), w188, ".txt" ("Substring")) -> (w190:string)
        n39 = local read "Transfer/Output - Gate"() -> (w135:u32)
        n40 = VISA Write(VISA resource name=w156, write buffer=":PAGE:CHAN:MODE SWE;" ("write buffer (\"\")"), error in (no error)=w155) -> (VISA resource name out=w153:refnum<visa-resource-name>, error out=w154:errorcluster)  [unwired: 1 out]
        n41 = String To Path(string=w190) -> (path=w185:path)
        n42 = case shown="\"d\", Default" w176 {
          tunnel: [w203 w204] -> w174
          frame "s" {
            w203 = u16 0 items=["Single", "Double"] ("sweep mode")
          }
          frame "d", Default {
            w204 = u16 1 items=["Single", "Double"] ("sweep mode")
          }
        }
        n43 = Fract/Exp String To Number(string=w175) -> (number=w160:dbl[])  [unwired: 3 in, 1 out]
        n44 = Index Array(array=w160, index #1=0 ("Index")) -> (element #1=w173:dbl, element #2=w172:dbl, element #3=w171:dbl)  [unwired: 2 in]
        n45 = Delete From Array(array=w160, length=3 ("Length"), index=0 ("Index")) -> (array with subset deleted=w158:dbl[])  [unwired: 1 out]
        n46 = Bundle By Name(cluster=w165, "Gate Start"=w173, "Gate Stop"=w172, "Gate Step (linear only)"=w171, "Gate Compliance"=w183, "Range mode"=w149, "Range"=w148) -> (w150:T3)
        n47 = Index Array(array=w158, index #1=0 ("Index")) -> (element #1=w168:dbl, element #2=w167:dbl, element #3=w166:dbl)  [unwired: 2 in]
        n48 = call <vilib>:"compatOverwrite.vi"("overwrite (F)"=TRUE) -> ("overwrite?"=w136:T7)
        n49 = Bundle By Name(cluster=w164, "Drain Start"=w168, "Drain Stop"=w167, "Drain Step"=w166, "Drain Compliance"=w184, "Range mode"=w147, "Range"=w146) -> (w151:T4)
        n50 = call "4155C Transfer v3.0.vi"("VISA resource name in"=w153, "Source/Common"=w132, 2:"Gate"=w150, 3:"Drain"=w151, 4:"Drain"=w133, "Timings"=w182, "error in (no error)"=w154, 7:"Probe 4"=w139, 8:"Gate"=w135, 9:"Probe 4"=w134, "sweep mode"=w174, "Panel Controls"=w138) -> ("VG"=w191:dbl[], "Outparams"=w144:T8, "VISA Resource Name out"=w180:refnum<visa-resource-name>, "IS"=w194:dbl[], "ID"=w193:dbl[], "IG"=w192:dbl[], "error out"=w181:errorcluster, "Probe 4"=w140:dbl[])  [unwired: 8 in]
        n51 = Unbundle By Name(w144) -> ("V2 Step"=w143:dbl, "V2 Start"=w142:dbl, "Number of points"=w141:i32)
        n52 = Open/Create/Replace File(file path (use dialog)=w185, error in=w181, operation (0:open)=w136) -> (refnum out=w200:refnum<file>, error out=w201:errorcluster)  [unwired: 3 in, 1 out]
        n53 = call "4155C Make Big 2d array.vi"("1D Var1"=w191, "1d IS"=w194, "1d ID"=w193, "1d IG"=w192, "1d SMU4"=w140, "SMU4"=w139, "VAR2 START"=w142, "Number of VAR2 steps"=w141, "VAR2 STEP"=w143, "VAR1 Name"="Vg", "Decimal places in header"=i8 1, "VAR2 Name"="Vd") -> ("Header array"=w196:string[], "Data array"=w197:dbl[][])  [unwired: 14 in]
        n54 = call "4155C Write array to file.vi"("Byte Stream File Refnum"=w200, "Header"=w196, "Data Array"=w197, "error in (no error)"=w201) -> ("dup refnum"=w198:refnum<file>, "error out"=w199:errorcluster)  [unwired: 1 in]
        n55 = Close File(refnum=w198, error in=w199) -> (error out=w179:errorcluster)  [unwired: 1 out]
      }
      frame "pulsedstressV" {
        w215 = 0
        n56 = Number To Decimal String(number=w264) -> (decimal integer string=w265:string)  [unwired: 1 in]
        n57 = local read "Pulsed Stress V - Drain"() -> (w206:u32)
        n58 = local read "Pulsed Stress V - Source/Common"() -> (w209:u32)
        n59 = Bundle By Name(cluster=w232, "Emergency Stop"=w268) -> (w234:T1)
        n60 = local read "Pulsed Stress V - Gate"() -> (w205:u32)
        n61 = Delete From Array(array=w256, index=0 ("Index")) -> (deleted portion=w254:string, array with subset deleted=w253:string[])  [unwired: 1 in]
        n62 = Concatenate Strings(w263, "-pulsedstressV-" ("Substring"), w265, ".txt" ("Substring")) -> (w267:string)
        n63 = VISA Write(VISA resource name=w247, write buffer=":PAGE:CHAN:MODE SWE;" ("write buffer (\"\")"), error in (no error)=w246) -> (VISA resource name out=w244:refnum<visa-resource-name>, error out=w245:errorcluster)  [unwired: 1 out]
        n64 = String To Path(string=w267) -> (path=w262:path)
        n65 = case shown="\"d\", Default" w254 {
          tunnel: [w277 w278] -> w252
          frame "s" {
            w277 = u16 0 items=["Single", "Double"] ("sweep mode")
          }
          frame "d", Default {
            w278 = u16 1 items=["Single", "Double"] ("sweep mode")
          }
        }
        n66 = Fract/Exp String To Number(string=w253) -> (number=w248:dbl[])  [unwired: 3 in, 1 out]
        n67 = local read "Pulsed Stress V - Probe 4"() -> (w207:u32)
        n68 = Index Array(array=w248, index #1=0 ("Index")) -> (element #1=w224:dbl, element #2=w223:dbl, element #3=w220:dbl, element #4=w219:dbl, element #5=w218:dbl, element #6=w222:dbl)  [unwired: 5 in]
        n69 = local read "Pulsed Stress V - Vextra"() -> (w208:u32)
        n70 = Bundle By Name(cluster=w221, "Pulse period"=w219, "Base voltage"=w220, "Pulse width"=w218) -> (w217:T5)
        n71 = Unbundle By Name(w217) -> ("Pulse period"=w225:dbl)
        n72 = Bundle By Name(cluster=w250, "Gate Start"=w223, "Gate Stop"=w224, "Gate Step (linear only)"=0, "Gate Compliance"=w260, "Range mode"=w240, "Range"=w239) -> (w241:T3)
        n73 = call <vilib>:"compatOverwrite.vi"("overwrite (F)"=TRUE) -> ("overwrite?"=w210:T7)
        n74 = Bundle By Name(cluster=w249, "Drain Start"=w222, "Drain Stop"=w215, "Drain Step"=w215, "Drain Compliance"=w261, "Range mode"=w238, "Range"=w237) -> (w242:T4)
        n75 = call "4155C PulsedStressV v3.0.vi"("VISA resource name in"=w244, "Gate"=w241, "Pulsed Stress V - Source/Common"=w209, "Drain"=w242, "Timings"=w217, "error in (no error)"=w245, "sweep mode"=w252, "Probe 4"=w233, "Pulsed Stress V - Drain"=w206, "Pulsed Stress V - Gate"=w205, "Panel Controls"=w234, "Pulsed Stress V - Probe 4"=w207, "Pulsed Stress V - Vextra"=w208) -> ("Outparams"=w235:T8, "VISA Resource Name out"=w258:refnum<visa-resource-name>, "ID"=w213:dbl[], "IG"=w211:dbl[], "error out"=w259:errorcluster)  [unwired: 2 in]
        n76 = Unbundle By Name(w235) -> ("Number of points"=w212:i32)  [unwired: 2 out]
        n77 = for {
          N: w212 -> [_]
          tunnel: [w274] -> w214 mode=indexing
          tunnel: w225 -> [w276]
          i -> [w275]
          n78 = Multiply(x=w276, y=w275) -> (x*y=w274:dbl)
        }
        n79 = Insert Into Array(array=dbl[][] [] ("Input Array"), new element=w214) -> (w226:dbl[][])  [unwired: 2 in]
        n80 = Insert Into Array(array=w226, new element=w213) -> (w231:dbl[][])  [unwired: 2 in]
        n81 = Insert Into Array(array=w231, new element=w211) -> (w230:dbl[][])  [unwired: 2 in]
        n82 = Transpose 2D Array(2D array=w230) -> (transposed array=w229:dbl[][])
        n83 = Open/Create/Replace File(file path (use dialog)=w262, error in=w259, operation (0:open)=w210) -> (refnum out=w271:refnum<file>, error out=w272:errorcluster)  [unwired: 3 in, 1 out]
        n84 = call "4155C Write array to file.vi"("Byte Stream File Refnum"=w271, "Header"=string[] ["Time /s", "Id /A", "Ig /A"], "Data Array"=w229, "error in (no error)"=w272) -> ("dup refnum"=w269:refnum<file>, "error out"=w270:errorcluster)  [unwired: 1 in]
        n85 = Close File(refnum=w269, error in=w270) -> (error out=w257:errorcluster)  [unwired: 1 out]
      }
      frame "transfer-fpp" {
        n86 = Number To Decimal String(number=w336) -> (decimal integer string=w337:string)  [unwired: 1 in]
        n87 = Bundle By Name(cluster=w312, "Emergency Stop"=w341) -> (w349:T6)
        n88 = local read "FPP - Source"() -> (w283:u32)
        n89 = Delete From Array(array=w327, index=0 ("Index")) -> (deleted portion=w325:string, array with subset deleted=w324:string[])  [unwired: 1 in]
        n90 = Concatenate Strings(w335, "-transferfpp-" ("Substring"), w337, ".txt" ("Substring")) -> (w339:string)
        n91 = local read "FPP - Drain"() -> (w280:u32)
        n92 = local read "FPP - Probe 1"() -> (w282:u32)
        n93 = VISA Write(VISA resource name=w304, write buffer=":PAGE:CHAN:MODE SWE;" ("write buffer (\"\")"), error in (no error)=w303) -> (VISA resource name out=w301:refnum<visa-resource-name>, error out=w302:errorcluster)  [unwired: 1 out]
        n94 = local read "FPP - Gate"() -> (w281:u32)
        n95 = String To Path(string=w339) -> (path=w334:path)
        n96 = case shown="\"d\", Default" w325 {
          tunnel: [w350 w351] -> w323
          frame "s" {
            w350 = u16 0 items=["Single", "Double"] ("sweep mode")
          }
          frame "d", Default {
            w351 = u16 1 items=["Single", "Double"] ("sweep mode")
          }
        }
        n97 = Fract/Exp String To Number(string=w324) -> (number=w308:dbl[])  [unwired: 3 in, 1 out]
        n98 = Index Array(array=w308, index #1=0 ("Index")) -> (element #1=w322:dbl, element #2=w321:dbl, element #3=w320:dbl)  [unwired: 2 in]
        n99 = local read "FPP - Probe 2"() -> (w279:u32)
        n100 = Delete From Array(array=w308, length=3 ("Length"), index=0 ("Index")) -> (array with subset deleted=w306:dbl[])  [unwired: 1 out]
        n101 = Bundle By Name(cluster=w314, "Gate Start"=w322, "Gate Stop"=w321, "Gate Step (linear only)"=w320, "Gate Compliance"=w332, "Range mode"=w297, "Range"=w296) -> (w298:T3)
        n102 = Index Array(array=w306, index #1=0 ("Index")) -> (element #1=w317:dbl, element #2=w316:dbl, element #3=w315:dbl)  [unwired: 2 in]
        n103 = call <vilib>:"compatOverwrite.vi"("overwrite (F)"=TRUE) -> ("overwrite?"=w284:T7)
        n104 = Bundle By Name(cluster=w313, "Drain Start"=w317, "Drain Stop"=w316, "Drain Step"=w315, "Drain Compliance"=w333, "Range mode"=w295, "Range"=w294) -> (w299:T4)
        n105 = call "4155C Transfer-FPP v3.0.vi"("VISA resource name in"=w301, "FPP - Source"=w283, "Gate"=w298, "Drain"=w299, "FPP - Drain"=w280, "Timings"=w331, "error in (no error)"=w302, "FPP - Gate"=w281, "FPP - Probe 1"=w282, "sweep mode"=w323, "FPP - Probe 2"=w279, "Panel Controls"=w349) -> ("VG"=w340:dbl[], "Outparams"=w292:T8, "VISA Resource Name out"=w329:refnum<visa-resource-name>, "Vprobe2"=w288:dbl[], "ID"=w287:dbl[], "IG"=w286:dbl[], "Vprobe1"=w285:dbl[], "error out"=w330:errorcluster)  [unwired: 8 in]
        n106 = Unbundle By Name(w292) -> ("V2 Step"=w291:dbl, "V2 Start"=w290:dbl, "Number of points"=w289:i32)
        n107 = Open/Create/Replace File(file path (use dialog)=w334, error in=w330, operation (0:open)=w284) -> (refnum out=w346:refnum<file>, error out=w347:errorcluster)  [unwired: 3 in, 1 out]
        n108 = call "4155C Make Big 2d array FPP.vi"("1D Var1"=w340, "1d ID"=w287, "1d Vp2"=w288, "1d IG"=w286, "1d Vp1"=w285, "VAR2 START"=w290, "Number of VAR2 steps"=w289, "VAR2 STEP"=w291, "VAR1 Name"="Vg", "Decimal places in header"=i8 1, "VAR2 Name"="Vd") -> ("Header array"=w342:string[], "Data array"=w343:dbl[][])  [unwired: 15 in]
        n109 = call "4155C Write array to file.vi"("Byte Stream File Refnum"=w346, "Header"=w342, "Data Array"=w343, "error in (no error)"=w347) -> ("dup refnum"=w344:refnum<file>, "error out"=w345:errorcluster)  [unwired: 1 in]
        n110 = Close File(refnum=w344, error in=w345) -> (error out=w328:errorcluster)  [unwired: 1 out]
      }
      frame "output" {
        n111 = local read "Stress V - Source/Common"() -> (w354:u32)
        n112 = Number To Decimal String(number=w404) -> (decimal integer string=w405:string)  [unwired: 1 in]
        n113 = local read "Transfer/Output - Probe 4"() -> (w355:u32)
        n114 = Bundle By Name(cluster=w380, "Emergency Stop"=w412) -> (w422:T6)
        n115 = local read "Transfer/Output - Drain"() -> (w352:u32)
        n116 = Delete From Array(array=w395, index=0 ("Index")) -> (deleted portion=w393:string, array with subset deleted=w392:string[])  [unwired: 1 in]
        n117 = Concatenate Strings(w403, "-output-" ("Substring"), w405, ".txt" ("Substring")) -> (w407:string)
        n118 = local read "Transfer/Output - Gate"() -> (w353:u32)
        n119 = VISA Write(VISA resource name=w371, write buffer=":PAGE:CHAN:MODE SWE;" ("write buffer (\"\")"), error in (no error)=w368) -> (VISA resource name out=w370:refnum<visa-resource-name>, error out=w369:errorcluster)  [unwired: 1 out]
        n120 = String To Path(string=w407) -> (path=w402:path)
        n121 = case shown="\"d\", Default" w393 {
          tunnel: [w423 w424] -> w391
          frame "s" {
            w423 = u16 0 items=["Single", "Double"] ("sweep mode")
          }
          frame "d", Default {
            w424 = u16 1 items=["Single", "Double"] ("sweep mode")
          }
        }
        n122 = Fract/Exp String To Number(string=w392) -> (number=w374:dbl[])  [unwired: 3 in, 1 out]
        n123 = Index Array(array=w374, index #1=0 ("Index")) -> (element #1=w390:dbl, element #2=w389:dbl, element #3=w388:dbl)  [unwired: 2 in]
        n124 = Delete From Array(array=w374, length=3 ("Length"), index=0 ("Index")) -> (array with subset deleted=w373:dbl[])  [unwired: 1 out]
        n125 = Bundle By Name(cluster=w382, "Gate Start"=w390, "Gate Stop"=w389, "Gate Step (linear only)"=w388, "Gate Compliance"=w400, "Range mode"=w366, "Range"=w365) -> (w421:T3)
        n126 = Index Array(array=w373, index #1=0 ("Index")) -> (element #1=w385:dbl, element #2=w384:dbl, element #3=w383:dbl)  [unwired: 2 in]
        n127 = call <vilib>:"compatOverwrite.vi"("overwrite (F)"=TRUE) -> ("overwrite?"=w356:T7)
        n128 = Bundle By Name(cluster=w381, "Drain Start"=w385, "Drain Stop"=w384, "Drain Step"=w383, "Drain Compliance"=w401, "Range mode"=w364, "Range"=w367) -> (w420:T4)
        n129 = call "4155C Output v3.0.vi"("VISA resource name in"=w370, "Source/Common"=w354, 2:"Gate"=w421, 3:"Drain"=w420, 4:"Drain"=w352, "Timings"=w399, "error in (no error)"=w369, 7:"Probe 4"=w358, 8:"Gate"=w353, 9:"Probe 4"=w355, "sweep mode"=w391, "Panel controls"=w422) -> ("VD"=w408:dbl[], "Outparams"=w361:T8, "VISA Resource Name out"=w397:refnum<visa-resource-name>, "IS"=w411:dbl[], "ID"=w410:dbl[], "IG"=w409:dbl[], "error out"=w398:errorcluster, "Probe 4"=w357:dbl[])  [unwired: 8 in]
        n130 = Unbundle By Name(w361) -> ("V2 Step"=w362:dbl, "V2 Start"=w360:dbl, "Number of points"=w359:i32)
        n131 = Open/Create/Replace File(file path (use dialog)=w402, error in=w398, operation (0:open)=w356) -> (refnum out=w417:refnum<file>, error out=w418:errorcluster)  [unwired: 3 in, 1 out]
        n132 = call "4155C Make Big 2d array.vi"("1D Var1"=w408, "1d IS"=w411, "1d ID"=w410, "1d IG"=w409, "1d SMU4"=w357, "SMU4"=w358, "VAR2 START"=w360, "Number of VAR2 steps"=w359, "VAR2 STEP"=w362, "VAR1 Name"="Vd", "Decimal places in header"=i8 1, "VAR2 Name"="Vg") -> ("Header array"=w413:string[], "Data array"=w414:dbl[][])  [unwired: 14 in]
        n133 = call "4155C Write array to file.vi"("Byte Stream File Refnum"=w417, "Header"=w413, "Data Array"=w414, "error in (no error)"=w418) -> ("dup refnum"=w415:refnum<file>, "error out"=w416:errorcluster)  [unwired: 1 in]
        n134 = Close File(refnum=w415, error in=w416) -> (error out=w396:errorcluster)  [unwired: 1 out]
      }
      frame "output-fpp" {
        n135 = Number To Decimal String(number=w481) -> (decimal integer string=w482:string)  [unwired: 1 in]
        n136 = Bundle By Name(cluster=w457, "Emergency Stop"=w485) -> (w495:T6)
        n137 = local read "FPP - Probe 1"() -> (w429:u32)
        n138 = Delete From Array(array=w472, index=0 ("Index")) -> (deleted portion=w470:string, array with subset deleted=w469:string[])  [unwired: 1 in]
        n139 = Concatenate Strings(w480, "-outputfpp-" ("Substring"), w482, ".txt" ("Substring")) -> (w484:string)
        n140 = local read "FPP - Gate"() -> (w426:u32)
        n141 = local read "FPP - Source"() -> (w425:u32)
        n142 = local read "FPP - Drain"() -> (w427:u32)
        n143 = VISA Write(VISA resource name=w448, write buffer=":PAGE:CHAN:MODE SWE;" ("write buffer (\"\")"), error in (no error)=w445) -> (VISA resource name out=w447:refnum<visa-resource-name>, error out=w446:errorcluster)  [unwired: 1 out]
        n144 = String To Path(string=w484) -> (path=w479:path)
        n145 = case shown="\"d\", Default" w470 {
          tunnel: [w496 w497] -> w468
          frame "s" {
            w496 = u16 0 items=["Single", "Double"] ("sweep mode")
          }
          frame "d", Default {
            w497 = u16 1 items=["Single", "Double"] ("sweep mode")
          }
        }
        n146 = Fract/Exp String To Number(string=w469) -> (number=w451:dbl[])  [unwired: 3 in, 1 out]
        n147 = Index Array(array=w451, index #1=0 ("Index")) -> (element #1=w467:dbl, element #2=w466:dbl, element #3=w465:dbl)  [unwired: 2 in]
        n148 = local read "FPP - Probe 2"() -> (w428:u32)
        n149 = Delete From Array(array=w451, length=3 ("Length"), index=0 ("Index")) -> (array with subset deleted=w450:dbl[])  [unwired: 1 out]
        n150 = Bundle By Name(cluster=w459, "Gate Start"=w467, "Gate Stop"=w466, "Gate Step (linear only)"=w465, "Gate Compliance"=w477, "Range mode"=w443, "Range"=w442) -> (w494:T3)
        n151 = Index Array(array=w450, index #1=0 ("Index")) -> (element #1=w462:dbl, element #2=w461:dbl, element #3=w460:dbl)  [unwired: 2 in]
        n152 = call <vilib>:"compatOverwrite.vi"("overwrite (F)"=TRUE) -> ("overwrite?"=w430:T7)
        n153 = Bundle By Name(cluster=w458, "Drain Start"=w462, "Drain Stop"=w461, "Drain Step"=w460, "Drain Compliance"=w478, "Range mode"=w441, "Range"=w444) -> (w493:T4)
        n154 = call "4155C Output-FPP v3.0.vi"("VISA resource name in"=w447, "FPP - Source"=w425, "Gate"=w494, "Drain"=w493, "FPP - Drain"=w427, "Timings"=w476, "error in (no error)"=w446, "FPP - Gate"=w426, "FPP - Probe 1"=w429, "sweep mode"=w468, "FPP - Probe 2"=w428, "Panel controls"=w495) -> ("VD"=w435:dbl[], "Outparams"=w438:T8, "VISA Resource Name out"=w474:refnum<visa-resource-name>, "Vprobe2"=w434:dbl[], "ID"=w433:dbl[], "IG"=w432:dbl[], "Vprobe1"=w431:dbl[], "error out"=w475:errorcluster)  [unwired: 8 in]
        n155 = Unbundle By Name(w438) -> ("V2 Step"=w439:dbl, "V2 Start"=w437:dbl, "Number of points"=w436:i32)
        n156 = Open/Create/Replace File(file path (use dialog)=w479, error in=w475, operation (0:open)=w430) -> (refnum out=w490:refnum<file>, error out=w491:errorcluster)  [unwired: 3 in, 1 out]
        n157 = call "4155C Make Big 2d array FPP.vi"("1D Var1"=w435, "1d ID"=w433, "1d Vp2"=w434, "1d IG"=w432, "1d Vp1"=w431, "VAR2 START"=w437, "Number of VAR2 steps"=w436, "VAR2 STEP"=w439, "VAR1 Name"="Vd", "Decimal places in header"=i8 1, "VAR2 Name"="Vg") -> ("Header array"=w486:string[], "Data array"=w487:dbl[][])  [unwired: 15 in]
        n158 = call "4155C Write array to file.vi"("Byte Stream File Refnum"=w490, "Header"=w486, "Data Array"=w487, "error in (no error)"=w491) -> ("dup refnum"=w488:refnum<file>, "error out"=w489:errorcluster)  [unwired: 1 in]
        n159 = Close File(refnum=w488, error in=w489) -> (error out=w473:errorcluster)  [unwired: 1 out]
      }
      frame "itime" {
        n160 = Delete From Array(array=w500, index=1) -> (deleted portion=w499:string)  [unwired: 1 in, 1 out]
        n161 = Delete From Array(array=w500, index=0 ("Index")) -> (deleted portion=w513:string)  [unwired: 1 in, 1 out]
        n162 = Fract/Exp String To Number(string=w499) -> (number=w498:dbl)  [unwired: 3 in, 1 out]
        n163 = case shown="\"s\"" w513 {
          tunnel: w512 -> [w518 w520 w524]
          tunnel: [w517 w519 w523] -> w505
          tunnel: w498 -> [w515 _ w522]
          frame "s" {
            w516 = u32 0 items=["short  ", "medium  ", "long  "] ("integration time 2")
            n164 = Bundle By Name(cluster=w518, "integration time"=w516, "Short/Long integration time"=w515) -> (w517:T5)
          }
          frame "m", Default {
            w521 = u32 1 items=["short  ", "medium  ", "long  "] ("integration time 2")
            n165 = Bundle By Name(cluster=w520, "integration time"=w521) -> (w519:T5)
          }
          frame "l" {
            w525 = u32 2 items=["short  ", "medium  ", "long  "] ("integration time 2")
            n166 = Bundle By Name(cluster=w524, "integration time"=w525, "Short/Long integration time"=w522) -> (w523:T5)
          }
        }
      }
      frame "pulsed" {
        n167 = Delete From Array(array=w538, index=0 ("Index")) -> (deleted portion=w539:string, array with subset deleted=w526:string[])  [unwired: 1 in]
        n168 = case shown="\"on\", Default" w539 {
          tunnel: w537 -> [w549 w552]
          tunnel: [w548 w551] -> w530
          tunnel: w526 -> [w546 _]
          frame "on", Default {
            w547 = u16 1 items=["Continuous", "Pulsed"] ("sweep method")
            n169 = Fract/Exp String To Number(string=w546) -> (number=w544:dbl[])  [unwired: 3 in, 1 out]
            n170 = Index Array(array=w544, index #1=0 ("Index")) -> (element #1=w543:dbl, element #2=w542:dbl, element #3=w541:dbl)  [unwired: 2 in]
            n171 = Bundle By Name(cluster=w549, "sweep method"=w547, "Pulse period"=w543, "Base voltage"=w542, "Pulse width"=w541) -> (w548:T5)
          }
          frame "off" {
            w550 = u16 0 items=["Continuous", "Pulsed"] ("sweep method")
            n172 = Bundle By Name(cluster=w552, "sweep method"=w550) -> (w551:T5)
          }
        }
      }
      frame "gaterangemode" {
        n173 = Delete From Array(array=w563, index=0 ("Index")) -> (deleted portion=w564:string)  [unwired: 1 in, 1 out]
        n174 = case shown="\"f\"" w564 {
          tunnel: [w566 w567 w568] -> w553
          frame "a", Default {
            w566 = u16 0 items=["Auto", "Limited", "Fixed"] ("Gate Range\nmode 2")
          }
          frame "f" {
            w567 = u16 2 items=["Auto", "Limited", "Fixed"] ("Gate Range\nmode 2")
          }
          frame "l" {
            w568 = u16 1 items=["Auto", "Limited", "Fixed"] ("Gate Range\nmode 2")
          }
        }
      }
      frame "gaterange" {
        (unwired) u8 11 items=["10fA  ", "100fA  ", "1nA  ", "10nA", "100nA", "1uA", "10uA", "100uA", "1mA", "10mA", "100mA", "1A"] ("Gate Range 2")
        n175 = Delete From Array(array=w586, index=0 ("Index")) -> (deleted portion=w576:string)  [unwired: 1 in, 1 out]
        n176 = Scan Value(string=w576, format string="") -> (value=w574:dbl)  [unwired: 1 in, 1 out]
        n177 = Logarithm Base 10(1:w574) -> (0:w573:dbl)
        n178 = Round To Nearest(number=w573) -> (nearest integer value=w572:dbl)
        n179 = Add(x=w572, y=11.0) -> (x+y=w570:dbl)
        n180 = To Unsigned Byte Integer(number=w570) -> (unsigned 8bit integer=w569:u8)
      }
      frame "drainrange" {
        (unwired) u8 11 items=["10fA  ", "100fA  ", "1nA  ", "10nA", "100nA", "1uA", "10uA", "100uA", "1mA", "10mA", "100mA", "1A"] ("Gate Range 2")
        n181 = Delete From Array(array=w605, index=0 ("Index")) -> (deleted portion=w596:string)  [unwired: 1 in, 1 out]
        n182 = Scan Value(string=w596, format string="") -> (value=w594:dbl)  [unwired: 1 in, 1 out]
        n183 = Logarithm Base 10(1:w594) -> (0:w593:dbl)
        n184 = Round To Nearest(number=w593) -> (nearest integer value=w592:dbl)
        n185 = Add(x=w592, y=11.0) -> (x+y=w590:dbl)
        n186 = To Unsigned Byte Integer(number=w590) -> (unsigned 8bit integer=w589:u8)
      }
      frame "drainrangemode" {
        n187 = Delete From Array(array=w617, index=0 ("Index")) -> (deleted portion=w618:string)  [unwired: 1 in, 1 out]
        n188 = case shown="\"f\"" w618 {
          tunnel: [w620 w621 w622] -> w607
          frame "a", Default {
            w620 = u16 0 items=["Auto", "Limited", "Fixed"] ("Gate Range\nmode 2")
          }
          frame "f" {
            w621 = u16 2 items=["Auto", "Limited", "Fixed"] ("Gate Range\nmode 2")
          }
          frame "l" {
            w622 = u16 1 items=["Auto", "Limited", "Fixed"] ("Gate Range\nmode 2")
          }
        }
      }
      frame "Error", Default {
      }
      frame "logfile" {
        n189 = Number To Decimal String(number=w663) -> (decimal integer string=w667:string)  [unwired: 1 in]
        n190 = Concatenate Strings(w665, "logfile" ("Substring"), w667, ".txt" ("Substring")) -> (w662:string)
        n191 = String To Path(string=w662) -> (path=w635:path)
        n192 = Unbundle(w661) -> ("integration time"=w660:u32, "Short/Long integration time"=w659:dbl, "hold time (sec)"=w658:dbl, "delay time (sec)"=w657:dbl, "Step Time (0 disables)"=w656:dbl, "sweep method"=w655:u16, "Pulse period"=w654:dbl, "Base voltage"=w653:dbl, "Pulse width"=w652:dbl)
        n193 = Build Array(w660, w659, w658, w657, w656, w655, w654, w653, w652, w646, w647, w648, w649, w650, w651) -> (w639:dbl[])
        n194 = Insert Into Array(array=dbl[][] [] ("Input Array"), new element=w639) -> (w638:dbl[][])  [unwired: 2 in]
        n195 = call <vilib>:"compatOverwrite.vi"("overwrite (F)"=TRUE) -> ("overwrite?"=w633:T7)
        n196 = Open/Create/Replace File(file path (use dialog)=w635, error in=w637, operation (0:open)=w633) -> (refnum out=w643:refnum<file>, error out=w642:errorcluster)  [unwired: 3 in, 1 out]
        n197 = call "4155C Write array to file.vi"("Byte Stream File Refnum"=w643, "Header"=string[] ["Int Time", "Short/Long Itime", "Hold time", "Delay time", "Step time", "Sweep method", "Pulse period", "Base Voltage", "Pulse width", "Drain compliance", "Gate compliance", "Gate range mode", "Gate range", "S/D range mode", "S/D range"], "Data Array"=w638, "error in (no error)"=w642) -> ("dup refnum"=w645:refnum<file>, "error out"=w644:errorcluster)  [unwired: 1 in]
        n198 = Close File(refnum=w645, error in=w644) -> (error out=w636:errorcluster)  [unwired: 1 out]
      }
      frame "sample" {
        n199 = Number To Decimal String(number=w720) -> (decimal integer string=w719:string)  [unwired: 1 in]
        n200 = local read "Sample - Source/Common"() -> (w669:u32)
        n201 = Fract/Exp String To Number(string=w716) -> (number=w676:dbl[])  [unwired: 3 in, 1 out]
        n202 = local read "Sample - Gate"() -> (w672:u32)
        n203 = Concatenate Strings(w694, "-sample-" ("Substring"), w719, ".txt" ("Substring")) -> (w717:string)
        n204 = local read "Sample - Drain"() -> (w671:u32)
        n205 = String To Path(string=w717) -> (path=w698:path)
        n206 = Index Array(array=w676, index=0 ("Index")) -> (element=w714:dbl)
        n207 = Index Array(array=w676, index=2 ("Index")) -> (element=w710:dbl)
        n208 = Index Array(array=w676, index=3 ("Index")) -> (element=w679:dbl)
        n209 = Index Array(array=w676, index=4 ("Index")) -> (element=w675:dbl)
        n210 = Index Array(array=w676, index=1 ("Index")) -> (element=w711:dbl)
        n211 = local read "Sample - Probe 4"() -> (w670:u32)
        n212 = call "4155C Config Sampling Measurements v3.0.vi"("VISA session"=w723, "Num Points"=w710, "Sample - Drain"=w671, "Display on/off"=TRUE, "Gate Compliance"=w695, "Sampling interval"=w675, "Sample - Source/Common"=w669, "Sample - Probe 4"=w670, "Drain Compliance"=w721, "error in (no error)"=w722, "Timings"=w685, "Sample - Gate"=w672, "Sample time"=w679) -> ("dup VISA resource name"=w725:refnum<visa-resource-name>, "error out"=w724:errorcluster)  [unwired: 1 in]
        n213 = call "4155C Take Sample v3.0.vi"("VISA resource name in"=w725, "Emergency Stop"=w691, "Sample - Gate"=w672, "Vg"=w714, "Sample - Drain"=w671, "Vd"=w711, "error in (no error)"=w724) -> ("Time"=w704:dbl[], "VISA Resource Name out"=w687:refnum<visa-resource-name>, "Ig"=w700:dbl[], "Id"=w727:dbl[], "Is"=w726:dbl[], "error out"=w689:errorcluster)  [unwired: 3 in]
        n214 = Insert Into Array(array=dbl[][] [] ("Input Array"), new element=w704) -> (w703:dbl[][])  [unwired: 2 in]
        n215 = Insert Into Array(array=w703, new element=w700) -> (w702:dbl[][])  [unwired: 2 in]
        n216 = Insert Into Array(array=w702, new element=w727) -> (w701:dbl[][])  [unwired: 2 in]
        n217 = VISA Write(VISA resource name=w687, write buffer=":DISP ON" ("write buffer (\"\")"), error in (no error)=w689) -> (VISA resource name out=w686:refnum<visa-resource-name>, error out=w688:errorcluster)  [unwired: 1 out]
        n218 = Insert Into Array(array=w701, new element=w726) -> (w693:dbl[][])  [unwired: 2 in]
        n219 = Transpose 2D Array(2D array=w693) -> (transposed array=w692:dbl[][])
        n220 = call <vilib>:"compatOverwrite.vi"("overwrite (F)"=TRUE) -> ("overwrite?"=w673:T7)
        n221 = Open/Create/Replace File(file path (use dialog)=w698, error in=w688, operation (0:open)=w673) -> (refnum out=w707:refnum<file>, error out=w706:errorcluster)  [unwired: 3 in, 1 out]
        n222 = call "4155C Write array to file.vi"("Byte Stream File Refnum"=w707, "Header"=string[] ["Time /s", "Ig /A", "Id /A", "Is /A"], "Data Array"=w692, "error in (no error)"=w706) -> ("dup refnum"=w709:refnum<file>, "error out"=w708:errorcluster)  [unwired: 1 in]
        n223 = Close File(refnum=w709, error in=w708) -> (error out=w696:errorcluster)  [unwired: 1 out]
      }
      frame "samplei" {
        n224 = local read "Sample I - Probe 4 (Disabled)"() -> (w731:u32)
        n225 = Number To Decimal String(number=w782) -> (decimal integer string=w781:string)  [unwired: 1 in]
        n226 = Fract/Exp String To Number(string=w778) -> (number=w744:dbl[])  [unwired: 3 in, 1 out]
        n227 = local read "Sample I - Source/Common"() -> (w728:u32)
        n228 = Concatenate Strings(w760, "-samplei-" ("Substring"), w781, ".txt" ("Substring")) -> (w779:string)
        n229 = local read "Sample I - Drain/Gate"() -> (w730:u32)
        n230 = String To Path(string=w779) -> (path=w763:path)
        n231 = Index Array(array=w744, index=4 ("Index")) -> (element=w738:dbl)
        n232 = Index Array(array=w744, index=3 ("Index")) -> (element=w739:dbl)
        n233 = Index Array(array=w744, index=1 ("Index")) -> (element=w741:dbl)
        n234 = Index Array(array=w744, index=0 ("Index")) -> (element=w742:dbl)
        n235 = Index Array(array=w744, index=2 ("Index")) -> (element=w740:dbl)
        n236 = local read "Sample I - Probe 3 (Disabled)"() -> (w729:u32)
        n237 = call "4155C Config SamplingI Measurements v3.0.vi"("VISA session"=w785, "Num Points"=w741, "Sample I - Probe 3 (Disabled)"=w729, "Display on/off"=TRUE, "Sample I - Source/Common"=w728, "Sample I - Drain/Gate"=w730, "Sampling interval"=w739, "error in (no error)"=w784, "Timings"=w752, "Sample I - Probe 4 (Disabled)"=w731, "Sample time"=w740) -> ("dup VISA resource name"=w787:refnum<visa-resource-name>, "error out"=w786:errorcluster)  [unwired: 3 in]
        n238 = call "4155C Take SampleI v3.0.vi"("Sample I - Drain/Gate"=w730, "Emergency Stop"=w757, "error in (no error)"=w786, "Idg 2"=w742, "Vdg compliance 2"=w738, "VISA resource name in"=w787) -> ("error out"=w755:errorcluster, "Idg"=w789:dbl[], "Vdg"=w765:dbl[], "VISA Resource Name out"=w753:refnum<visa-resource-name>, "Is"=w788:dbl[], "Time"=w769:dbl[])
        n239 = Insert Into Array(array=dbl[][] [] ("Input Array"), new element=w769) -> (w768:dbl[][])  [unwired: 2 in]
        n240 = Insert Into Array(array=w768, new element=w765) -> (w767:dbl[][])  [unwired: 2 in]
        n241 = Insert Into Array(array=w767, new element=w789) -> (w766:dbl[][])  [unwired: 2 in]
        n242 = VISA Write(VISA resource name=w753, write buffer=":DISP ON" ("write buffer (\"\")"), error in (no error)=w755) -> (VISA resource name out=w737:refnum<visa-resource-name>, error out=w754:errorcluster)  [unwired: 1 out]
        n243 = Insert Into Array(array=w766, new element=w788) -> (w759:dbl[][])  [unwired: 2 in]
        n244 = Transpose 2D Array(2D array=w759) -> (transposed array=w758:dbl[][])
        n245 = call <vilib>:"compatOverwrite.vi"("overwrite (F)"=TRUE) -> ("overwrite?"=w732:T7)
        n246 = Open/Create/Replace File(file path (use dialog)=w763, error in=w754, operation (0:open)=w732) -> (refnum out=w772:refnum<file>, error out=w771:errorcluster)  [unwired: 3 in, 1 out]
        n247 = call "4155C Write array to file.vi"("Byte Stream File Refnum"=w772, "Header"=string[] ["Time /s", "Vdg /V", "Idg /A", "Is /A"], "Data Array"=w758, "error in (no error)"=w771) -> ("dup refnum"=w774:refnum<file>, "error out"=w773:errorcluster)  [unwired: 1 in]
        n248 = Close File(refnum=w774, error in=w773) -> (error out=w735:errorcluster)  [unwired: 1 out]
        n249 = VISA Write(VISA resource name=w737, write buffer=";:PAGE:SCON:STAN OFF;:PAGE:CHAN:VSU2:DIS;" ("write buffer (\"\")"), error in (no error)=w735) -> (VISA resource name out=w733:refnum<visa-resource-name>, error out=w734:errorcluster)  [unwired: 1 out]
      }
      frame "#" {
        n250 = VISA Write(VISA resource name=w794, write buffer=":DISP ON" ("write buffer (\"\")"), error in (no error)=w793) -> (VISA resource name out=w792:refnum<visa-resource-name>, error out=w791:errorcluster)  [unwired: 1 out]
      }
      frame "stressV" {
        n251 = Number To Decimal String(number=w845) -> (decimal integer string=w844:string)  [unwired: 1 in]
        n252 = Fract/Exp String To Number(string=w841) -> (number=w813:dbl[])  [unwired: 3 in, 1 out]
        n253 = Concatenate Strings(w828, "-stressV-" ("Substring"), w844, ".txt" ("Substring")) -> (w842:string)
        n254 = local read "Stress V - Drain"() -> (w805:u32)
        n255 = String To Path(string=w842) -> (path=w832:path)
        n256 = Index Array(array=w813, index=3 ("Index")) -> (element=w810:dbl)
        n257 = Index Array(array=w813, index=1 ("Index")) -> (element=w808:dbl)
        n258 = Index Array(array=w813, index=0 ("Index")) -> (element=w807:dbl)
        n259 = Index Array(array=w813, index=4 ("Index")) -> (element=w812:dbl)
        n260 = Index Array(array=w813, index=2 ("Index")) -> (element=w809:dbl)
        n261 = local read "Stress V - Source/Common"() -> (w803:u32)
        n262 = local read "Stress V - Gate"() -> (w804:u32)
        n263 = call "4155C Config V Stress v3.0.vi"("Display on/off"=TRUE, "Stress V - Gate"=w804, "Stress V - Drain"=w805, "Stress V - Source/Common"=w803, "IG compliance"=w809, "ID compliance"=w810, "error in (no error)"=w847, "VG"=w807, "VD"=w808, "VISA session"=w848) -> ("error out"=w849:errorcluster, "dup VISA resource name"=w850:refnum<visa-resource-name>)
        n264 = call "4155C Apply Stress.vi"("error in (no error)"=w849, "Duration"=w812, "Emergency Stop"=w827, "VISA resource name in"=w850) -> ("error out"=w825:errorcluster, "VISA Resource Name out"=w823:refnum<visa-resource-name>)
        n265 = VISA Write(VISA resource name=w823, write buffer=":DISP ON" ("write buffer (\"\")"), error in (no error)=w825) -> (VISA resource name out=w822:refnum<visa-resource-name>, error out=w824:errorcluster)  [unwired: 1 out]
        n266 = call <vilib>:"compatOverwrite.vi"("overwrite (F)"=TRUE) -> ("overwrite?"=w806:T7)
        n267 = Open/Create/Replace File(file path (use dialog)=w832, error in=w824, operation (0:open)=w806) -> (refnum out=w835:refnum<file>, error out=w834:errorcluster)  [unwired: 3 in, 1 out]
        n268 = call "4155C Write array to file.vi"("Byte Stream File Refnum"=w835, "Header"=string[] ["V stress completed successfully", ""], "error in (no error)"=w834) -> ("dup refnum"=w837:refnum<file>, "error out"=w836:errorcluster)  [unwired: 2 in]
        n269 = Close File(refnum=w837, error in=w836) -> (error out=w830:errorcluster)  [unwired: 1 out]
      }
      frame "stressI" {
        n270 = Number To Decimal String(number=w888) -> (decimal integer string=w887:string)  [unwired: 1 in]
        n271 = Fract/Exp String To Number(string=w884) -> (number=w858:dbl[])  [unwired: 3 in, 1 out]
        n272 = Concatenate Strings(w871, "-stressI-" ("Substring"), w887, ".txt" ("Substring")) -> (w885:string)
        n273 = String To Path(string=w885) -> (path=w875:path)
        n274 = Index Array(array=w858, index=1 ("Index")) -> (element=w854:dbl)
        n275 = Index Array(array=w858, index=0 ("Index")) -> (element=w855:dbl)
        n276 = Index Array(array=w858, index=2 ("Index")) -> (element=w856:dbl)
        n277 = local read "Stress I - Drain/Gate"() -> (w852:u32)
        n278 = local read "Stress I - Source/Common"() -> (w851:u32)
        n279 = call "4155C Config I Stress v3.0.vi"("Stress I - Drain/Gate"=w852, "Stress I - Source/Common"=w851, "Display on/off"=TRUE, "error in (no error)"=w890, "VDG compliance"=w854, "IDG"=w855, "VISA session"=w891) -> ("error out"=w892:errorcluster, "dup VISA resource name"=w893:refnum<visa-resource-name>)  [unwired: 1 in]
        n280 = call "4155C Apply Stress.vi"("error in (no error)"=w892, "Duration"=w856, "Emergency Stop"=w870, "VISA resource name in"=w893) -> ("error out"=w868:errorcluster, "VISA Resource Name out"=w866:refnum<visa-resource-name>)
        n281 = VISA Write(VISA resource name=w866, write buffer=":DISP ON" ("write buffer (\"\")"), error in (no error)=w868) -> (VISA resource name out=w865:refnum<visa-resource-name>, error out=w867:errorcluster)  [unwired: 1 out]
        n282 = call <vilib>:"compatOverwrite.vi"("overwrite (F)"=TRUE) -> ("overwrite?"=w853:T7)
        n283 = Open/Create/Replace File(file path (use dialog)=w875, error in=w867, operation (0:open)=w853) -> (refnum out=w878:refnum<file>, error out=w877:errorcluster)  [unwired: 3 in, 1 out]
        n284 = call "4155C Write array to file.vi"("Byte Stream File Refnum"=w878, "Header"=string[] ["I stress completed successfully", ""], "error in (no error)"=w877) -> ("dup refnum"=w880:refnum<file>, "error out"=w879:errorcluster)  [unwired: 2 in]
        n285 = Close File(refnum=w880, error in=w879) -> (error out=w873:errorcluster)  [unwired: 1 out]
      }
      frame "vsu2pulse" {
        n286 = Number To Decimal String(number=w928) -> (decimal integer string=w927:string)  [unwired: 1 in]
        n287 = local read "VSU2 Stress - Source/Common"() -> (w894:u32)
        n288 = Fract/Exp String To Number(string=w924) -> (number=w899:dbl[])  [unwired: 3 in, 1 out]
        n289 = Concatenate Strings(w912, "-vsu2-" ("Substring"), w927, ".txt" ("Substring")) -> (w925:string)
        n290 = String To Path(string=w925) -> (path=w916:path)
        n291 = Index Array(array=w899, index=1 ("Index")) -> (element=w898:dbl)
        n292 = Index Array(array=w899, index=0 ("Index")) -> (element=w896:dbl)
        n293 = call "4155C Config VSU2 Stress v3.0.vi"("VISA session"=w931, "Display on/off"=TRUE, "VSU2"=w896, "error in (no error)"=w930, "VSU2 Stress - Source/Common"=w894) -> ("dup VISA resource name"=w933:refnum<visa-resource-name>, "error out"=w932:errorcluster)
        n294 = call "4155C Apply Stress.vi"("error in (no error)"=w932, "Duration"=w898, "Emergency Stop"=w911, "VISA resource name in"=w933) -> ("error out"=w909:errorcluster, "VISA Resource Name out"=w907:refnum<visa-resource-name>)
        n295 = VISA Write(VISA resource name=w907, write buffer=":DISP ON" ("write buffer (\"\")"), error in (no error)=w909) -> (VISA resource name out=w906:refnum<visa-resource-name>, error out=w908:errorcluster)  [unwired: 1 out]
        n296 = call <vilib>:"compatOverwrite.vi"("overwrite (F)"=TRUE) -> ("overwrite?"=w895:T7)
        n297 = Open/Create/Replace File(file path (use dialog)=w916, error in=w908, operation (0:open)=w895) -> (refnum out=w919:refnum<file>, error out=w918:errorcluster)  [unwired: 3 in, 1 out]
        n298 = call "4155C Write array to file.vi"("Byte Stream File Refnum"=w919, "Header"=string[] ["VSU2 pulse completed successfully", ""], "error in (no error)"=w918) -> ("dup refnum"=w921:refnum<file>, "error out"=w920:errorcluster)  [unwired: 2 in]
        n299 = Close File(refnum=w921, error in=w920) -> (error out=w914:errorcluster)  [unwired: 1 out]
      }
      frame "sample-fpp" {
        w946 = string[] ["Time /s", "Id VgVd /A", "Ig VgVd /A", "Vp1 VgVd /V", "Vp2 VgVd /V"] ("Header")
        w950 = "%d" ("format string")
        n300 = local read "FPP - Drain"() -> (w935:u32)
        n301 = local read "FPP - Source"() -> (w936:u32)
        n302 = local read "FPP - Probe 1"() -> (w937:u32)
        n303 = Number To Decimal String(number=w1000) -> (decimal integer string=w999:string)  [unwired: 1 in]
        n304 = Fract/Exp String To Number(string=w996) -> (number=w984:dbl[])  [unwired: 3 in, 1 out]
        n305 = Concatenate Strings(w990, "-samplefpp-" ("Substring"), w999, ".txt" ("Substring")) -> (w997:string)
        n306 = String To Path(string=w997) -> (path=w958:path)
        n307 = local read "FPP - Gate"() -> (w934:u32)
        n308 = Index Array(array=w984, index=0 ("Index")) -> (element=w944:dbl)
        n309 = Index Array(array=w984, index=1 ("Index")) -> (element=w943:dbl)
        n310 = local read "FPP - Probe 2"() -> (w938:u32)
        n311 = Index Array(array=w984, index=2 ("Index")) -> (element=w992:dbl)
        n312 = Index Array(array=w984, index=3 ("Index")) -> (element=w982:dbl)
        n313 = call "4155C Config Sampling Measurements FPP v3.0.vi"("VISA session"=w1003, "Gate Compliance"=w991, "FPP - Source"=w936, "FPP - Drain"=w935, "Drain Compliance"=w1001, "error in (no error)"=w1002, "Num Points"=w992, "Timings"=w989, "FPP - Gate"=w934, "FPP - Probe 1"=w937, "Vg"=w944, "Vd"=w943, "Display on/off"=TRUE, "Sample time"=w982, "FPP - Probe 2"=w938, "Standby"="Standby") -> ("dup VISA resource name"=w960:refnum<visa-resource-name>, "error out"=w959:errorcluster)  [unwired: 2 in]
        n314 = Number To Decimal String(number=w944) -> (decimal integer string=w970:string)  [unwired: 1 in]
        n315 = call "4155C Take Sample FPP.vi"("VISA resource name in"=w960, "error in (no error)"=w959, "Emergency Stop"=w961) -> ("Time"=w965:dbl[], "Vp1"=w975:dbl[], "VISA Resource Name out"=w941:refnum<visa-resource-name>, "Ig"=w963:dbl[], "Id"=w964:dbl[], "Vp2"=w973:dbl[], "error out"=w962:errorcluster)  [unwired: 10 in]
        n316 = Insert Into Array(array=dbl[][] [] ("Input Array"), new element=w965) -> (w979:dbl[][])  [unwired: 2 in]
        n317 = Number To Decimal String(number=w943) -> (decimal integer string=w968:string)  [unwired: 1 in]
        n318 = Insert Into Array(array=w979, new element=w964) -> (w978:dbl[][])  [unwired: 2 in]
        n319 = Concatenate Strings("(Vg = " ("Substring"), w970, "V, Vd = " ("Substring"), w968, "V)" ("Substring")) -> (w966:string)
        n320 = Insert Into Array(array=w978, new element=w963) -> (w977:dbl[][])  [unwired: 2 in]
        n321 = Insert Into Array(array=w977, new element=w975) -> (w974:dbl[][])  [unwired: 2 in]
        n322 = Insert Into Array(array=w974, new element=w973) -> (w942:dbl[][])  [unwired: 2 in]
        n323 = call <vilib>:"compatOverwrite.vi"("overwrite (F)"=TRUE) -> ("overwrite?"=w939:T7)
        n324 = Open/Create/Replace File(file path (use dialog)=w958, error in=w962, operation (0:open)=w939) -> (refnum out=w955:refnum<file>, error out=w956:errorcluster)  [unwired: 3 in, 1 out]
        n325 = Array To Spreadsheet String(array=w946, 3:w950) -> (spreadsheet string=w952:string)  [unwired: 1 in]
        n326 = Transpose 2D Array(2D array=w942) -> (transposed array=w972:dbl[][])
        n327 = Search and Replace String(replace all?=TRUE ("replace all? (F)"), input string=w952, search string="VgVd", replace string=w966) -> (result string=w948:string)  [unwired: 4 in, 3 out]
        n328 = Spreadsheet String To Array(format string=w950, spreadsheet string=w948, array type (2D Dbl)=w946) -> (array=w947:string[])  [unwired: 1 in]
        n329 = call "4155C Write array to file.vi"("Byte Stream File Refnum"=w955, "Header"=w947, "Data Array"=w972, "error in (no error)"=w956) -> ("dup refnum"=w953:refnum<file>, "error out"=w954:errorcluster)  [unwired: 1 in]
        n330 = Close File(refnum=w953, error in=w954) -> (error out=w940:errorcluster)  [unwired: 1 out]
      }
      frame "resample-fpp" {
        w1013 = string[] ["Time /s", "Id VgVd /A", "Ig VgVd /A", "Vp1 VgVd /V", "Vp2 VgVd /V"] ("Header")
        w1017 = "%d" ("format string")
        n331 = Number To Decimal String(number=w1059) -> (decimal integer string=w1058:string)  [unwired: 1 in]
        n332 = Fract/Exp String To Number(string=w1055) -> (number=w1006:dbl[])  [unwired: 3 in, 1 out]
        n333 = Concatenate Strings(w1051, "-resamplefpp-" ("Substring"), w1058, ".txt" ("Substring")) -> (w1056:string)
        n334 = String To Path(string=w1056) -> (path=w1025:path)
        n335 = Index Array(array=w1006, index=0 ("Index")) -> (element=w1012:dbl)
        n336 = Index Array(array=w1006, index=1 ("Index")) -> (element=w1011:dbl)
        n337 = Number To Decimal String(number=w1012) -> (decimal integer string=w1035:string)  [unwired: 1 in]
        n338 = call "4155C Take Sample FPP.vi"("VISA resource name in"=w1008, "error in (no error)"=w1007, "Emergency Stop"=w1026) -> ("Time"=w1030:dbl[], "Vp1"=w1040:dbl[], "VISA Resource Name out"=w1010:refnum<visa-resource-name>, "Ig"=w1028:dbl[], "Id"=w1029:dbl[], "Vp2"=w1038:dbl[], "error out"=w1027:errorcluster)  [unwired: 10 in]
        n339 = Insert Into Array(array=dbl[][] [] ("Input Array"), new element=w1030) -> (w1044:dbl[][])  [unwired: 2 in]
        n340 = Number To Decimal String(number=w1011) -> (decimal integer string=w1033:string)  [unwired: 1 in]
        n341 = Insert Into Array(array=w1044, new element=w1029) -> (w1043:dbl[][])  [unwired: 2 in]
        n342 = Concatenate Strings("(Vg = " ("Substring"), w1035, "V, Vd = " ("Substring"), w1033, "V)" ("Substring")) -> (w1031:string)
        n343 = Insert Into Array(array=w1043, new element=w1028) -> (w1042:dbl[][])  [unwired: 2 in]
        n344 = Insert Into Array(array=w1042, new element=w1040) -> (w1039:dbl[][])  [unwired: 2 in]
        n345 = Insert Into Array(array=w1039, new element=w1038) -> (w1005:dbl[][])  [unwired: 2 in]
        n346 = call <vilib>:"compatOverwrite.vi"("overwrite (F)"=TRUE) -> ("overwrite?"=w1004:T7)
        n347 = Open/Create/Replace File(file path (use dialog)=w1025, error in=w1027, operation (0:open)=w1004) -> (refnum out=w1022:refnum<file>, error out=w1023:errorcluster)  [unwired: 3 in, 1 out]
        n348 = Array To Spreadsheet String(array=w1013, 3:w1017) -> (spreadsheet string=w1019:string)  [unwired: 1 in]
        n349 = Transpose 2D Array(2D array=w1005) -> (transposed array=w1037:dbl[][])
        n350 = Search and Replace String(replace all?=TRUE ("replace all? (F)"), input string=w1019, search string="VgVd", replace string=w1031) -> (result string=w1015:string)  [unwired: 4 in, 3 out]
        n351 = Spreadsheet String To Array(format string=w1017, spreadsheet string=w1015, array type (2D Dbl)=w1013) -> (array=w1014:string[])  [unwired: 1 in]
        n352 = call "4155C Write array to file.vi"("Byte Stream File Refnum"=w1022, "Header"=w1014, "Data Array"=w1037, "error in (no error)"=w1023) -> ("dup refnum"=w1020:refnum<file>, "error out"=w1021:errorcluster)  [unwired: 1 in]
        n353 = Close File(refnum=w1020, error in=w1021) -> (error out=w1009:errorcluster)  [unwired: 1 out]
      }
    }
    n354 = local write "Lines left to run:"(w39) -> ()
    n355 = Empty String/Path?(string/path=w39) -> (empty?=w75:bool)
    n356 = Not(x=w75) -> (.not. x?=w74:bool)
  }
